vi "Main UI (standalone).vi"() -> ()   [LabVIEW 2015]
doc: "User interface for 64 pressure multiplexer system designed by Paul Nathan, 02/2016"
uses:
  Ctls/System status.ctl
  Ctls/Environmental state values.ctl
  Ctls/Inertial state values.ctl
  Ctls/AccelGyro constants.ctl
  Ctls/Pressure sensor constants.ctl
  Ctls/Cmd str.ctl
  Ctls/All state values (for datalog).ctl
  Ctls/Data values, Mode 0 (for datalog).ctl
  Ctls/Data values, Mode 1 (for datalog).ctl
panel:
  in  "Main tabs":enum32{"Startup & config.", "Datastream"}(tab)
  out "ASCII done":bool caption="Done"
  in  "Write ASCII datalog":bool
  in  "Datalog name (without extension)":string="Log001"
  in  "Write interval (s)":u32=10
  in  "Save data":bool
  in  "Datalog directory":path=path "C:/Datalogs"
  out "ACK 8":bool caption="ACK"
  out "ACK 7":bool caption="ACK"
  out "ACK 6":bool caption="ACK"
  out "AccelGyro constants":T1={"gyrRange"=125.0, "accRange"=2.0, "gx offset"=0.0, "gy offset"=0.0, "gz offset"=0.0, "ax offset"=0.0, "ay offset"=0.0, "az offset"=0.0, "axyz scale"=1.0} {"axyz scale" format="%#_4f"; "az offset" format="%#_4f"; "ay offset" format="%#_4f"; "ax offset" format="%#_4f"; "gz offset" format="%#_4f"; "gy offset" format="%#_4f"; "gx offset" format="%#_4f"; "gyrRange" format="%#_4f"; "accRange" format="%#_4f"}
  out "Faulty sensors":i32[](array[numeric])
  out "ACK 5":bool caption="ACK"
  in  "Stop UI":bool
  out "Active sensors":i32[](array[numeric])
  in  "Refresh sys. status":bool
  out "ACK 4":bool caption="ACK"
  in  "Apply settings 3":bool caption="Apply settings"
  in  "Gyro. rate (Hz)":u8(ring) items=["6.25", "12.5", "25", "50", "100", "200", "400", "800", "1600", "3200"]
  in  "Gyro. range (dps)":u8(ring) items=["+/- 125", "+/- 250", "+/- 500", "+/- 1000", "+/- 2000"]
  in  "Accel. rate (Hz)":u8(ring)=1 items=["3.125", "6.25", "12.5", "25", "50", "100", "200", "400", "800", "1600"]
  in  "Accel. range (g)":u8(ring) items=["+/- 2", "+/- 4", "+/- 8", "+/- 16"]
  out "Inertial state values":T2 {"w_z (dps)" format="%#_4f"; "a_y (g)" format="%#_4f"; "a_z (g)" format="%#_4f"; "w_y (dps)" format="%#_4f"; "a_x (g)" format="%#_4f"; "Sensor temp. (degC)" format="%#.2f"; "w_x (dps)" format="%#_4f"}
  out "Environmental state values":T3 {"Dew point (degC)" format="%#.2f"; "Density (kg/m^3)" format="%#.3f"; "Pressure alt. (m)" format="%#.2f"; "Density alt. (m)" format="%#.2f"; "Rel. Humidity (%)" format="%#.2f"; "P_atmos (Pa)" format="%#_6f"; "Sensor temp. (degC)" format="%#.2f"; "Thermistor (degC)" format="%#.2f"}
  out "System status":T4
  out "ACK 3":bool caption="ACK"
  in  "Apply settings 2":bool caption="Apply setting"
  in  "Max. num. sensors (override)":u8=64 max=64
  out "ACK 1":bool caption="ACK"
  in  "Env. period (ms)":i32=1000 min=0
  in  "Data mode":u8(ring) items=["P", "P & T"]
  out "ACK 2":bool caption="ACK"
  in  "Apply settings 1":bool caption="Apply settings"
  in  "Data rate (Hz)":dbl=100.0
  in  "Reset":bool
  in  "Main Power":bool
  in  "Serial port":refnum<visa-resource-name>="COM1"
  out "Error":errorcluster
  out "L_data (bytes)":u16
  out "Serial no.":u16 format="%04x"
  out "Active pressure sensor constants":T5[](array[typedef])
  in  "d.p":i16=4
  in  "Wait for HW trigger":bool
  out "Clock drift":bool
  in  "Display rate (Hz)":dbl=100.0 min=0.0
  in  "N samples":u32=1000
  in  "Finite samples":bool
  out "Sensor temperatures time trace (Mode \"P & T\" only)":sgl[][](graph)
  out "Pressures time trace":sgl[][](graph)
  in  "Stop streaming":bool
  in  "Start streaming":bool
  out "Stale samples flag":u8[][](graph)
  out "Samples acquired":u32
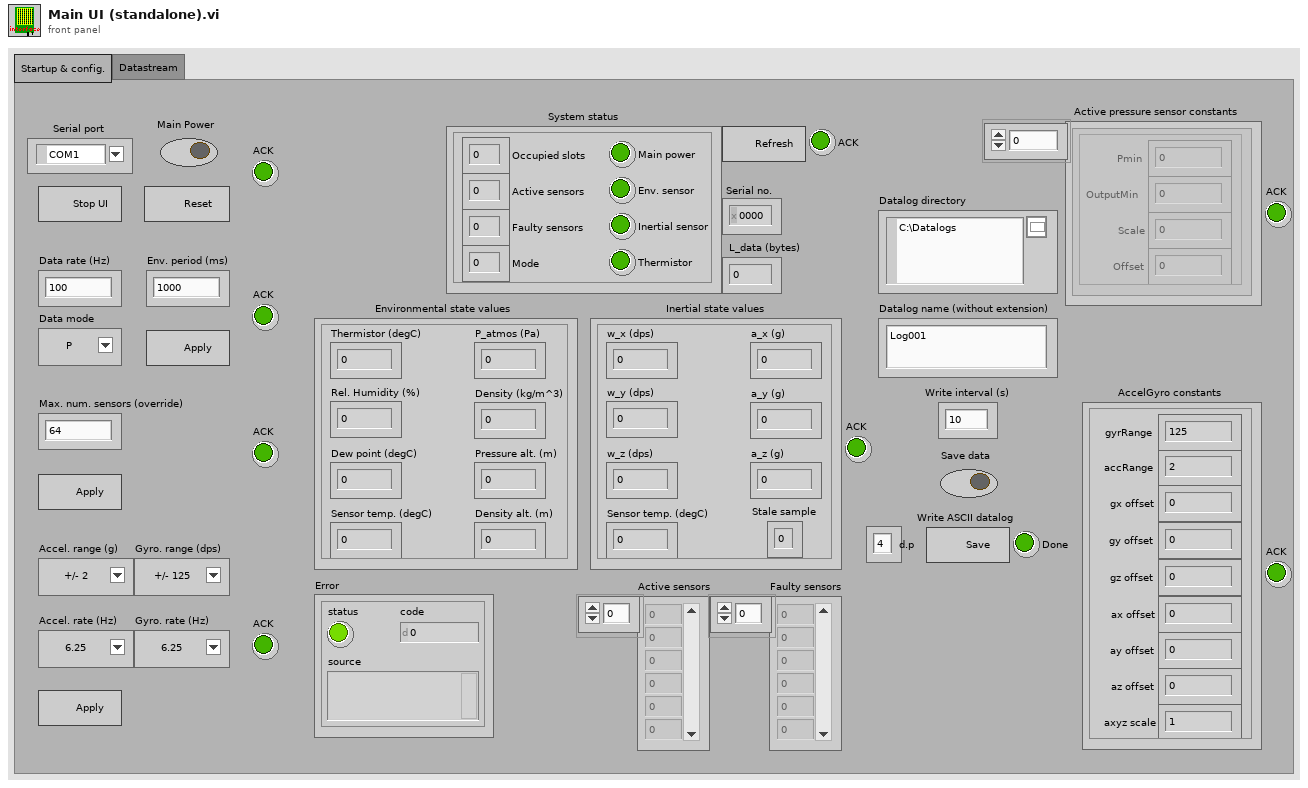
[diagram p1: front panel]
types:
  T1 = typedef "AccelGyro constants.ctl" = cluster{"gyrRange":sgl, "accRange":sgl, "gx offset":sgl, "gy offset":sgl, "gz offset":sgl, "ax offset":sgl, "ay offset":sgl, "az offset":sgl, "axyz scale":sgl}
  T2 = typedef "Inertial state values.ctl" = cluster{"w_x (dps)":sgl, "w_y (dps)":sgl, "w_z (dps)":sgl, "a_x (g)":sgl, "a_y (g)":sgl, "a_z (g)":sgl, "Stale sample":u8, "Sensor temp. (degC)":sgl}
  T3 = typedef "Environmental state values.ctl" = cluster{"Thermistor (degC)":sgl, "Sensor temp. (degC)":sgl, "P_atmos (Pa)":sgl, "Rel. Humidity (%)":sgl, "Density (kg/m^3)":sgl, "Dew point (degC)":sgl, "Pressure alt. (m)":sgl, "Density alt. (m)":sgl}
  T4 = typedef "System status.ctl" = cluster{"Main power":bool, "Occupied slots":u8, "Active sensors":u8, "Faulty sensors":u8, "Env. sensor":bool, "Inertial sensor":bool, "Thermistor":bool, "Mode":u8}
  T5 = typedef "Pressure sensor constants.ctl" = cluster{"Pmin":sgl, "OutputMin":sgl, "Scale":sgl, "Offset":sgl}
  T6 = typedef "Cmd str.ctl" = string
  T7 = typedef "All state values (for datalog).ctl" = cluster{"Time Stamp":timestamp, "dt (ms)":i32, "Environmental state values":T3, "Inertial state values":T2}
  T8 = typedef "Data values, Mode 1 (for datalog).ctl" = cluster{"Time Stamp":timestamp, "dt (us)":sgl, "dt_warn":u8, "Pressures":sgl[], "Die temps.":sgl[], "Statuses":u8[]}
  T9 = typedef "Data values, Mode 0 (for datalog).ctl" = cluster{"Time Stamp":timestamp, "dt (us)":sgl, "dt_warn":u8, "Pressures":sgl[], "Statuses":u8[]}
  T10 = enum8{"Enabled", "Disabled", "Disabled and Grayed Out"}
  T11 = typedef "EEPROM page.ctl" = cluster{"Pmin (Pa)":sgl, "Pmax (Pa)":sgl, "maxCount":u16, "minCount":u16, "Poffset (Pa)":sgl}
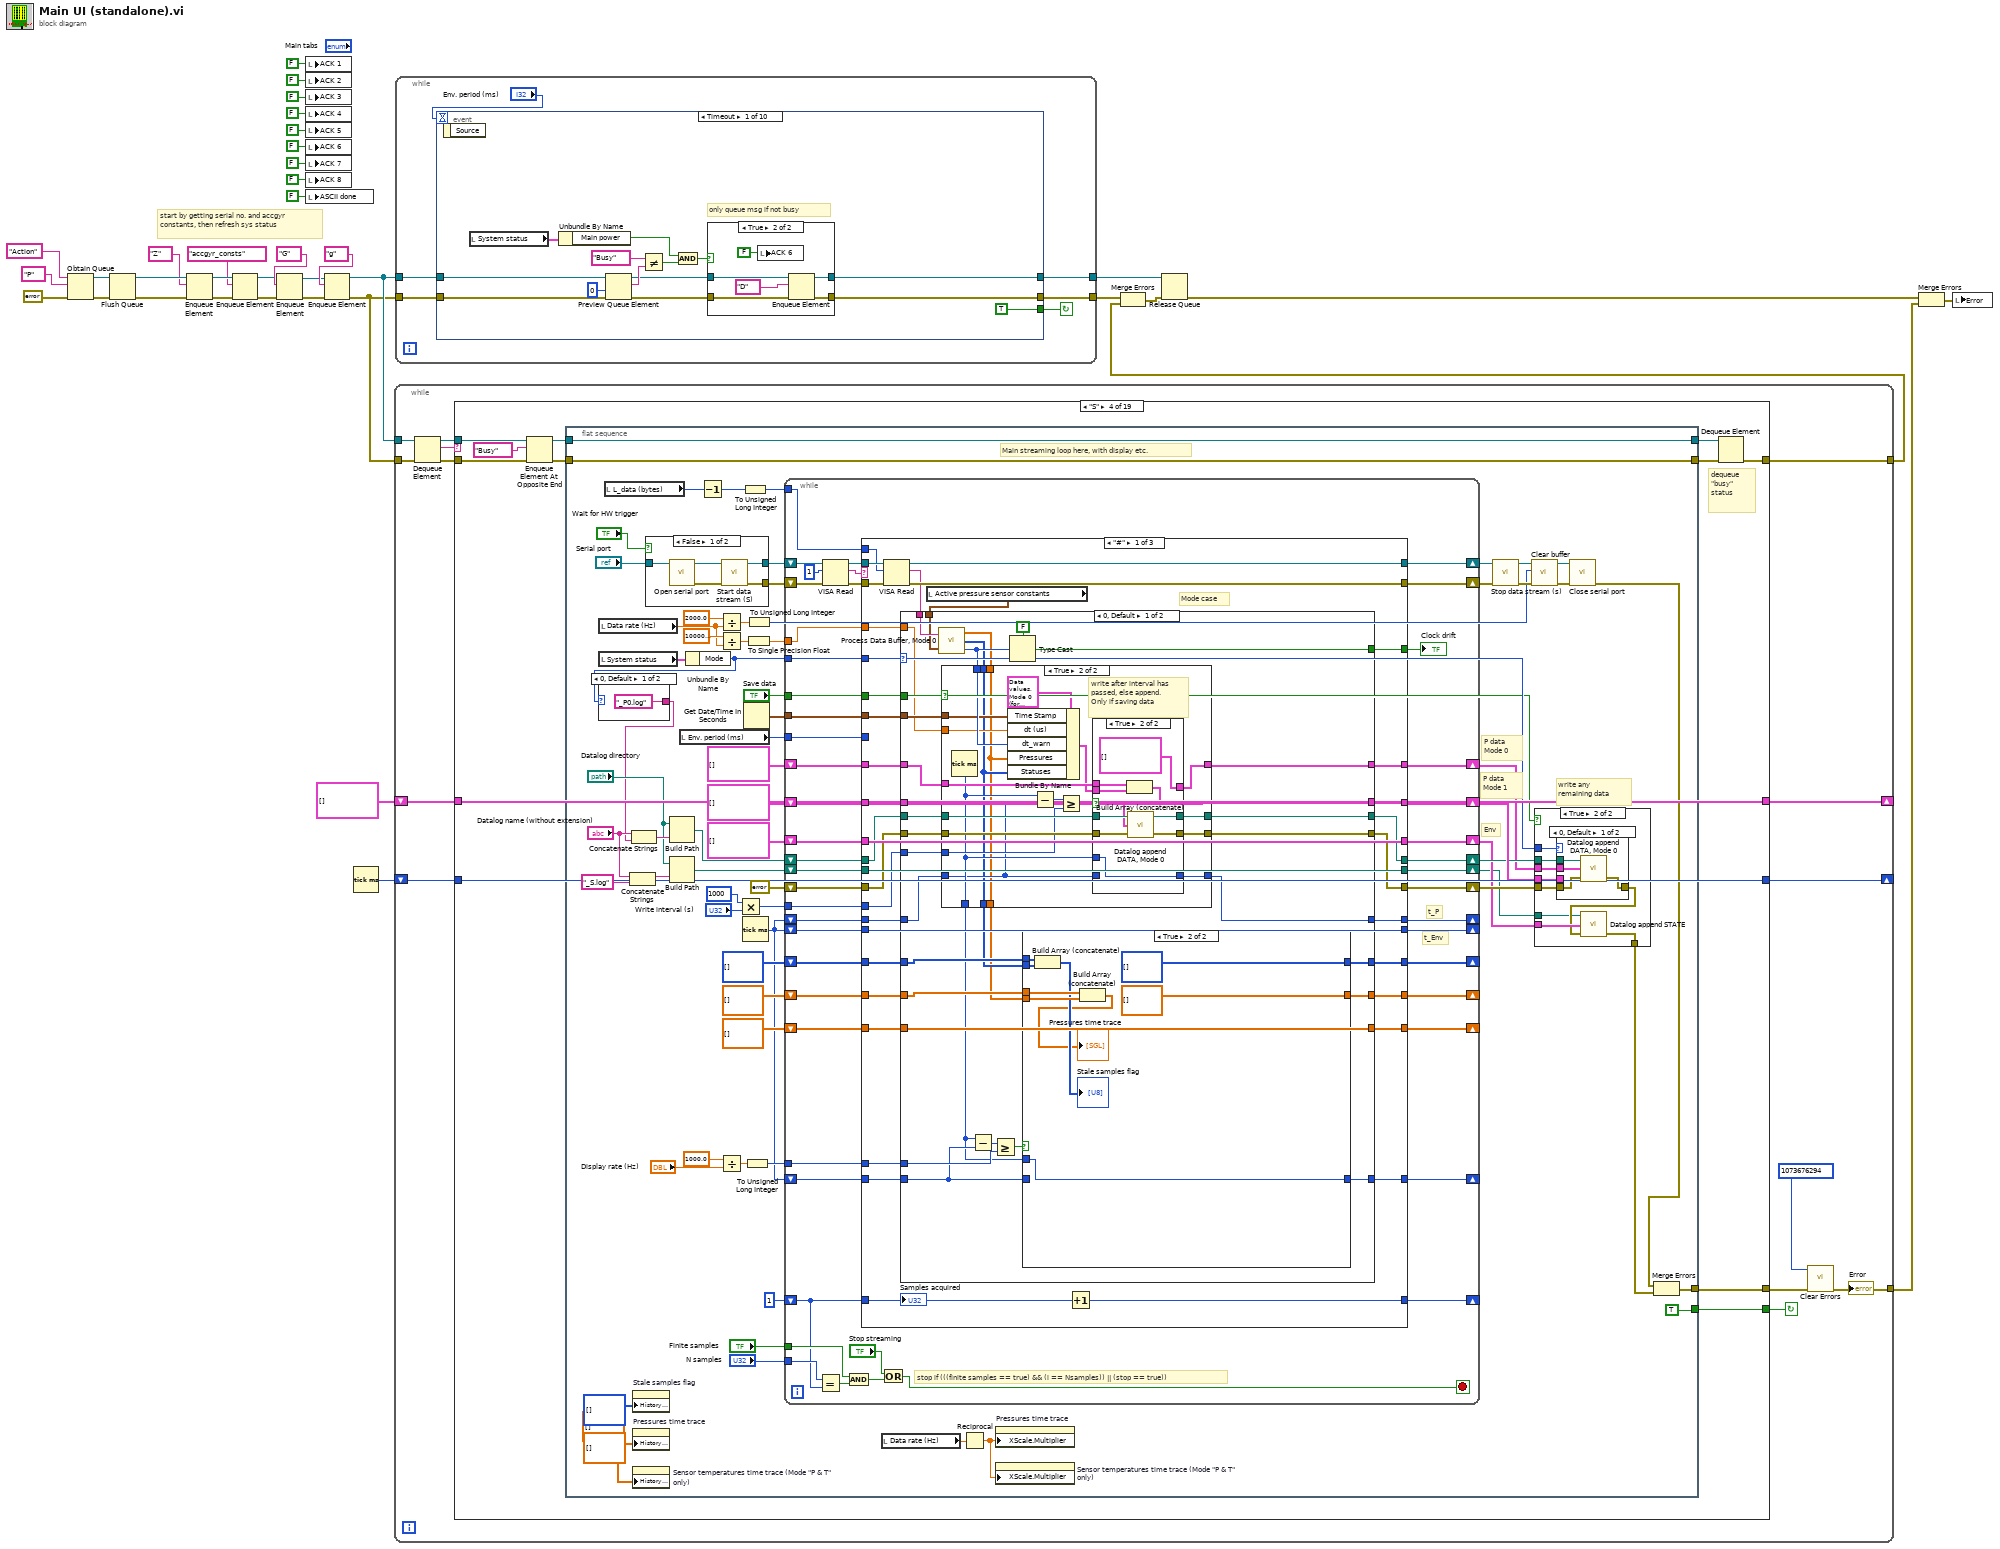
[diagram p0: block diagram]
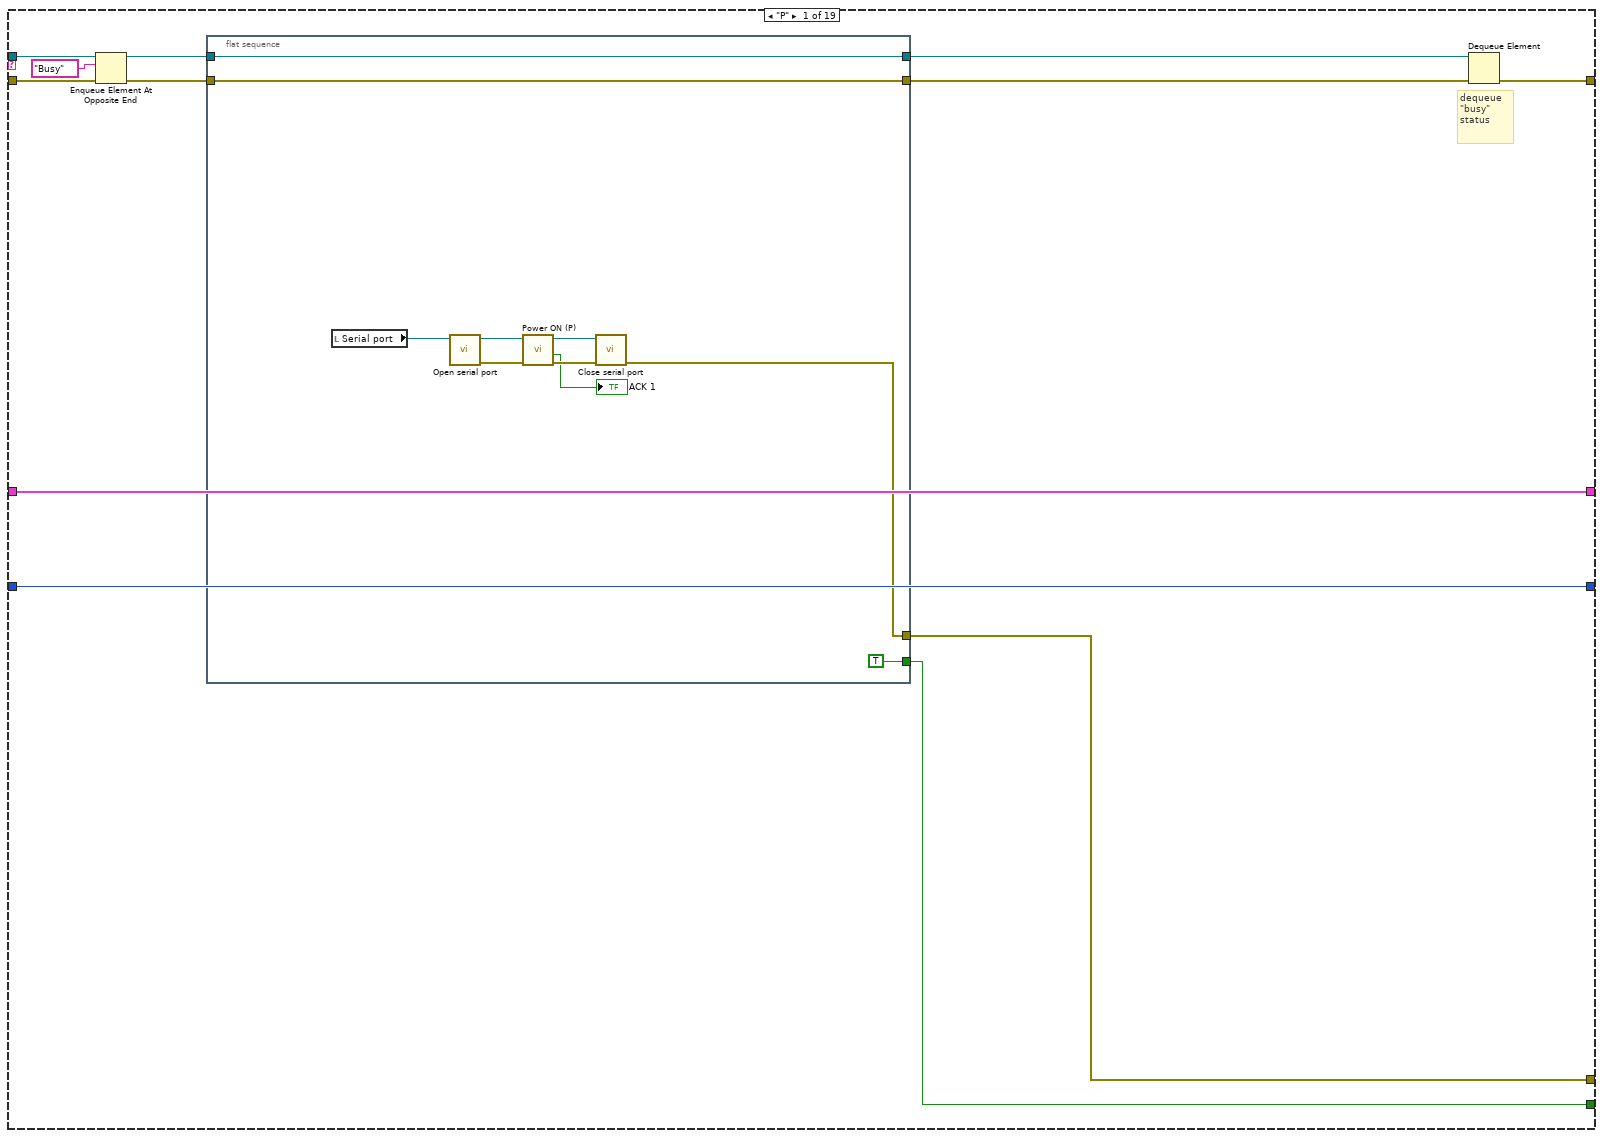
[diagram p2: hidden frame]
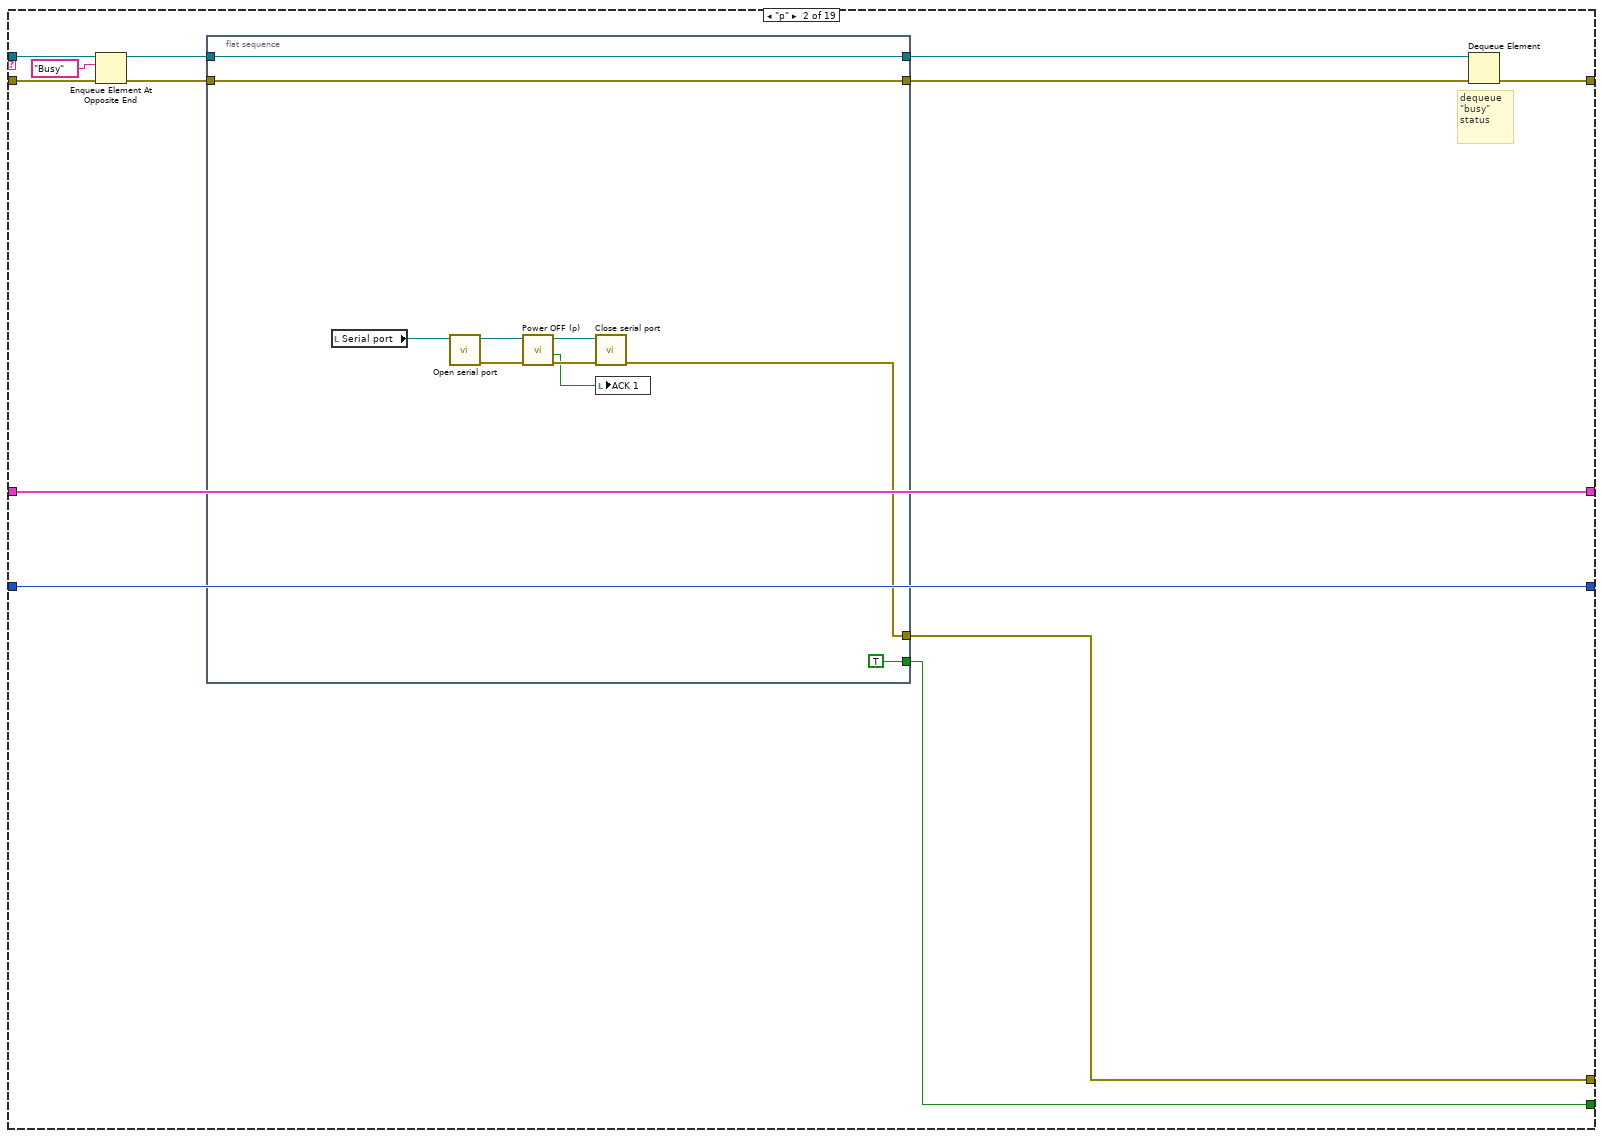
[diagram p3: hidden frame]
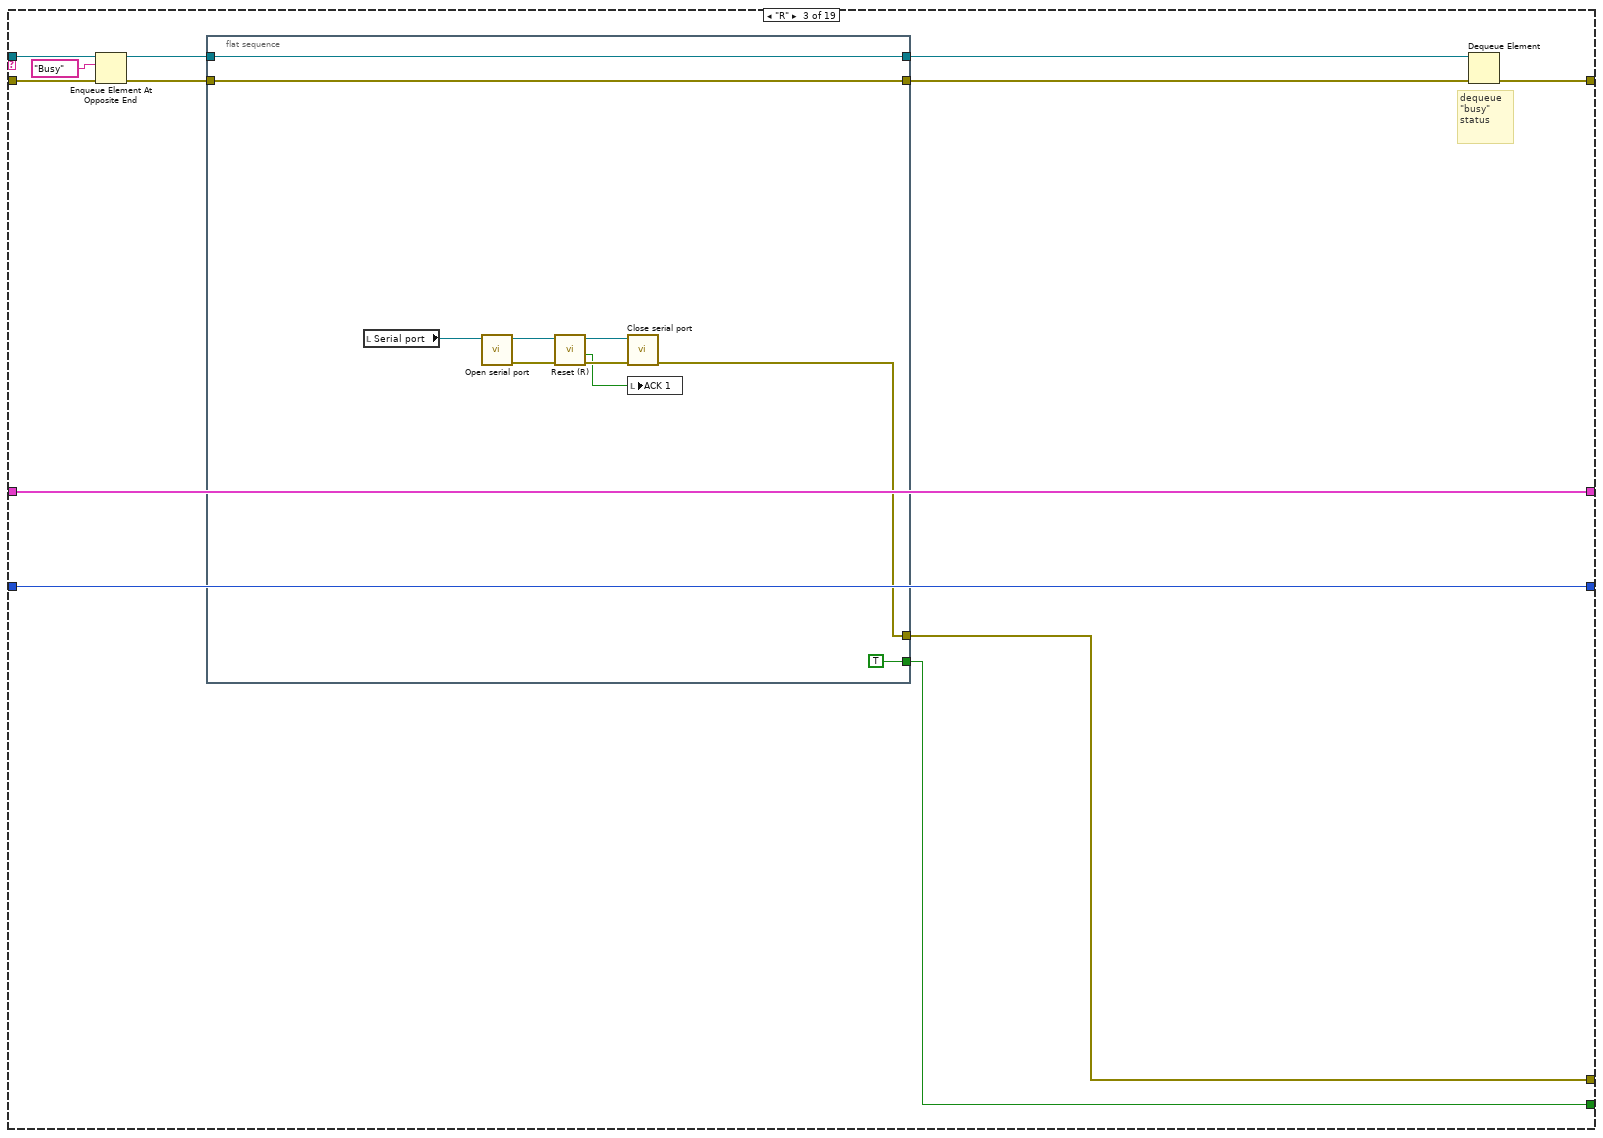
[diagram p4: hidden frame]
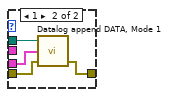
[diagram p6: hidden frame]
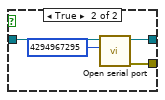
[diagram p7: hidden frame]
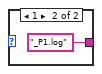
[diagram p8: hidden frame]
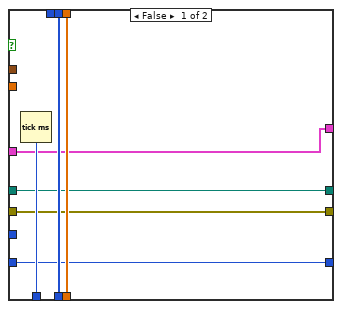
[diagram p9: hidden frame]
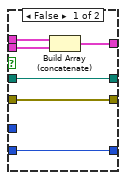
[diagram p10: hidden frame]
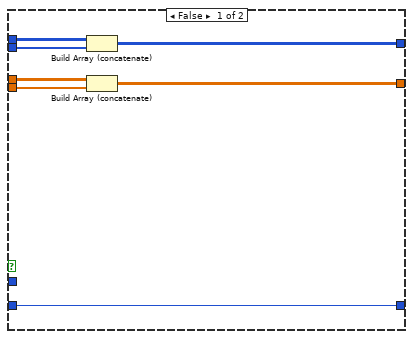
[diagram p11: hidden frame]
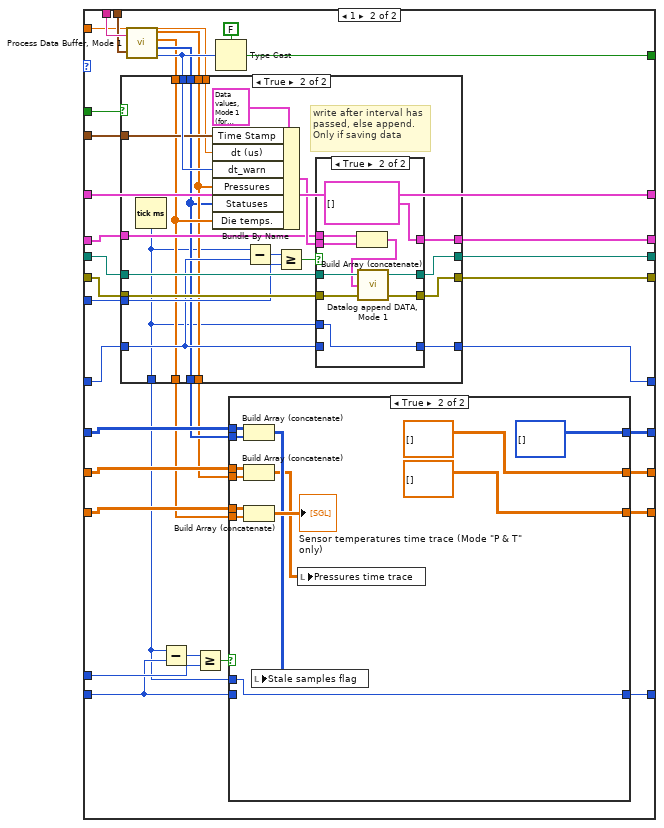
[diagram p12: hidden frame]
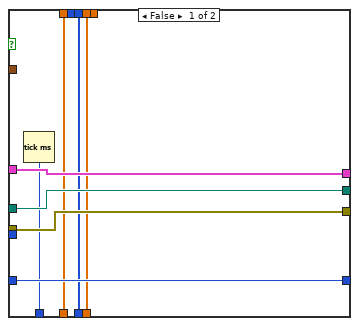
[diagram p13: hidden frame]
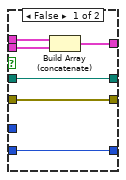
[diagram p14: hidden frame]
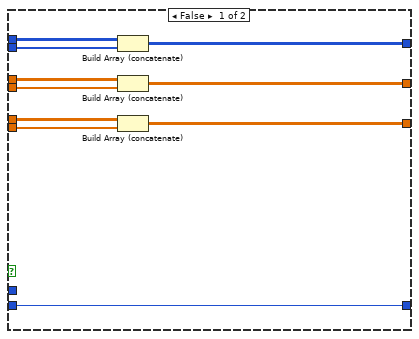
[diagram p15: hidden frame]
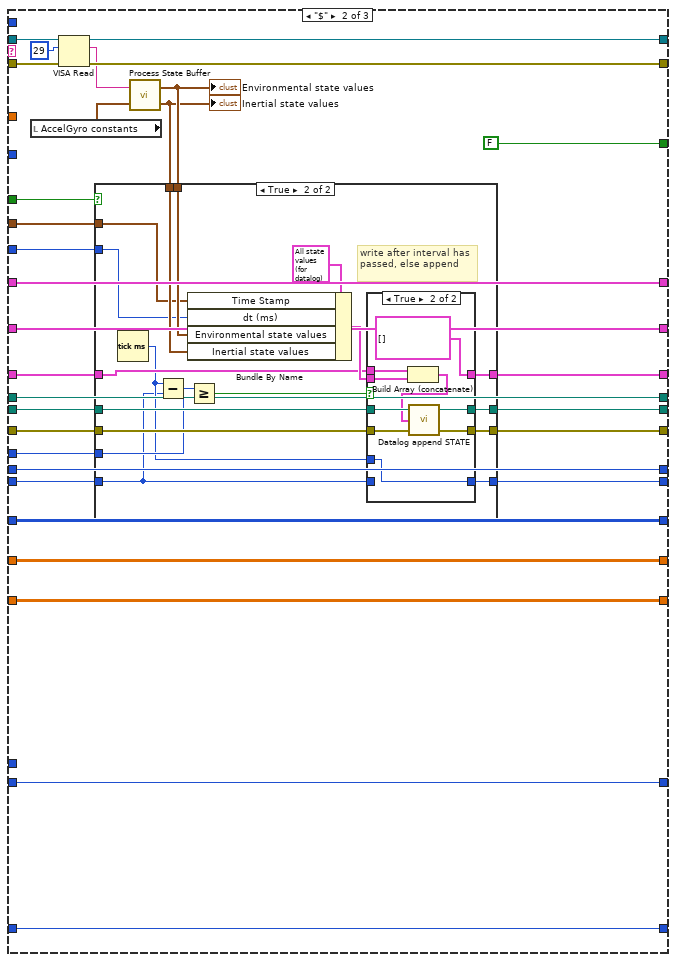
[diagram p16: hidden frame]
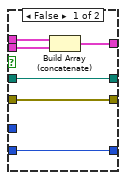
[diagram p18: hidden frame]
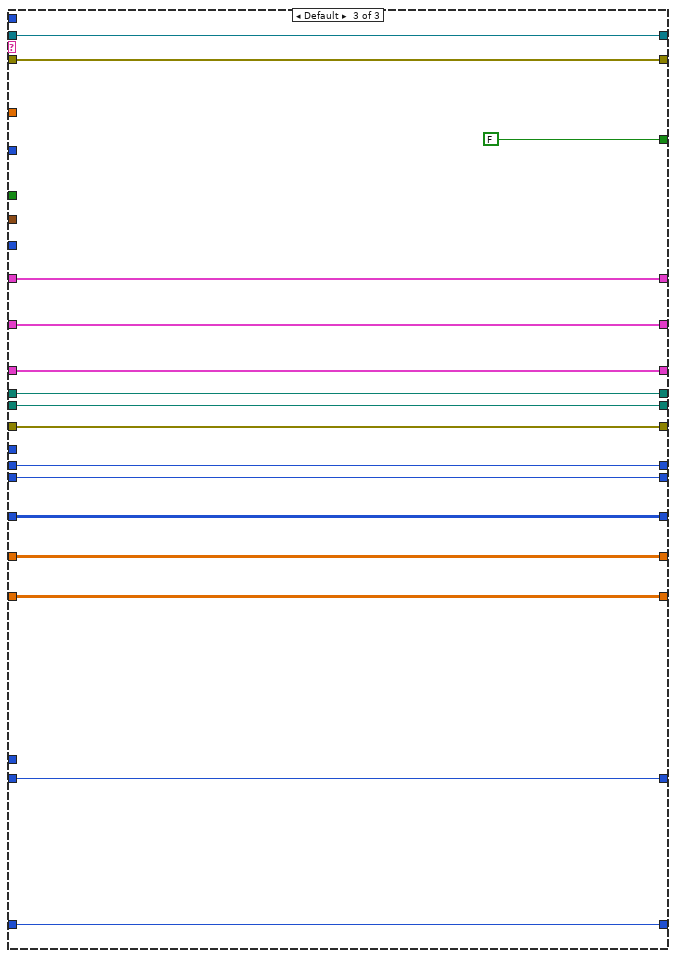
[diagram p19: hidden frame]
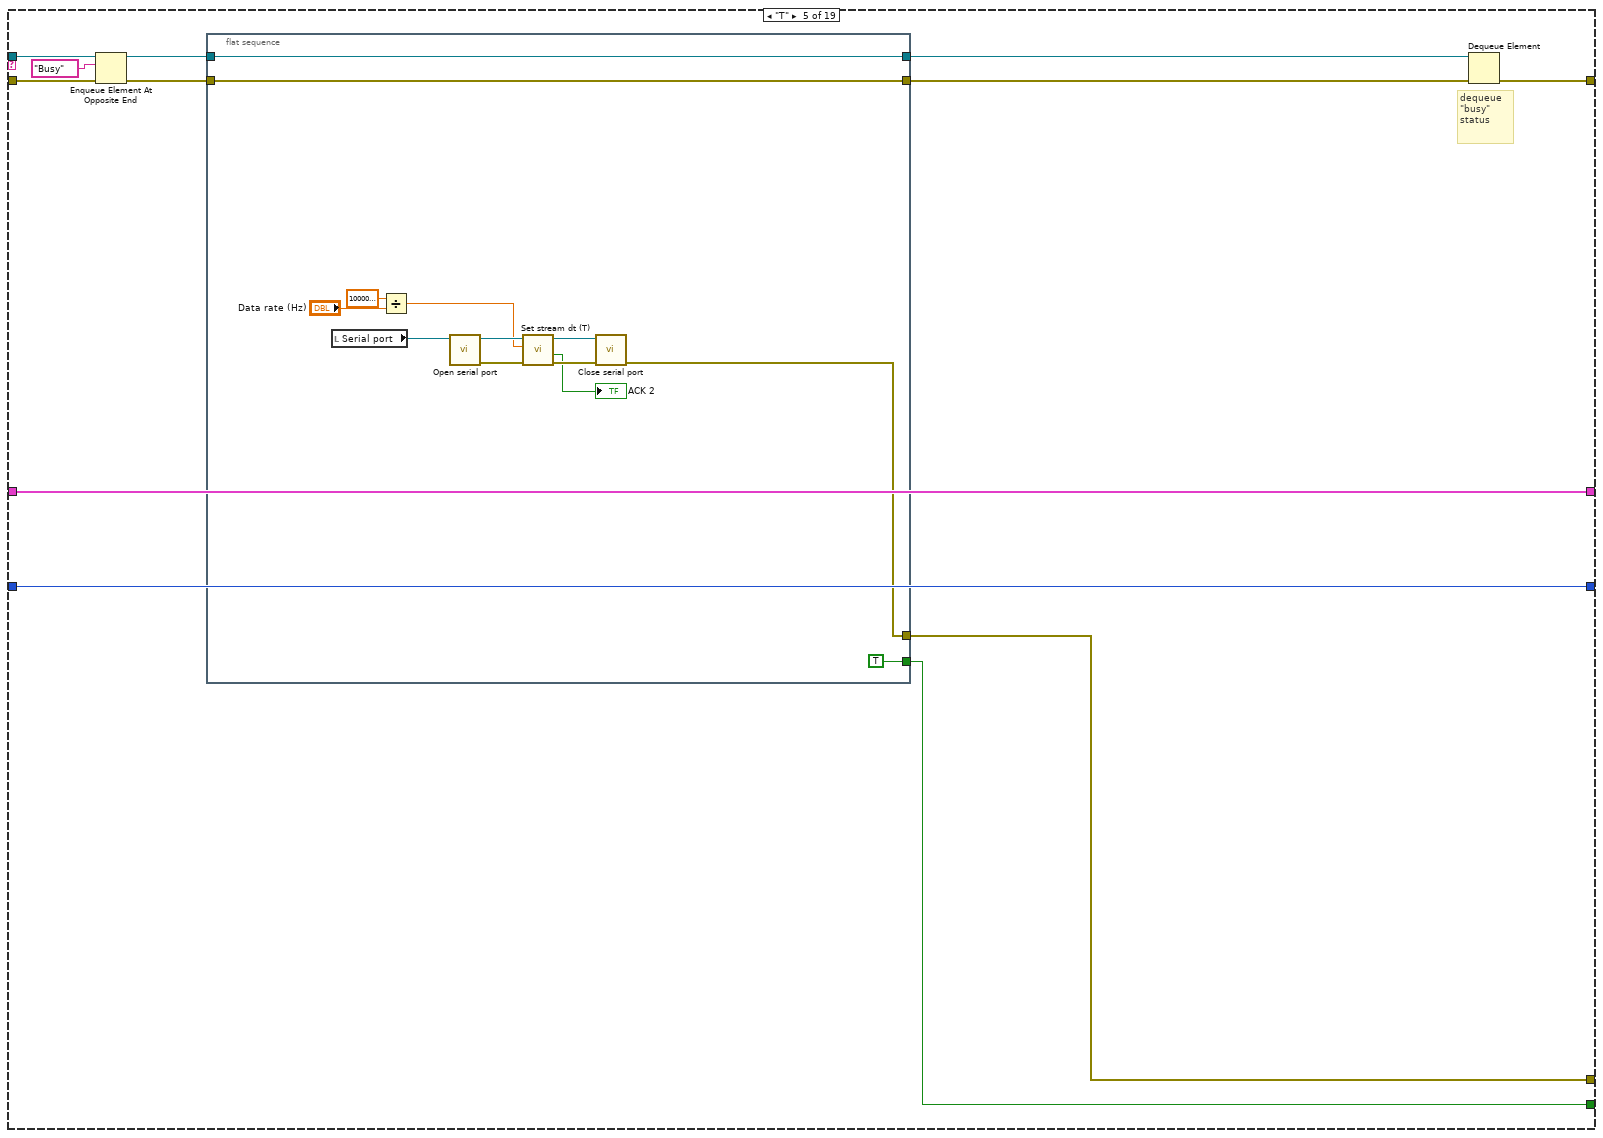
[diagram p20: hidden frame]
diagram:
  # "start by getting serial no. and accgyr constants, then refresh sys status"
  n1 = Obtain Queue(name (unnamed)="Action", element data type=T6 "P" ("Cmd"), error in (no error)=errorcluster {"status"=FALSE, "code"=0, "source"=""}) -> (queue out=w36:refnum<queue>, error out=w35:errorcluster)  [unwired: 2 in, 1 out]
  n2 = Flush Queue(queue=w36, error in (no error)=w35) -> (queue out=w28:refnum<queue>, error out=w27:errorcluster)  [unwired: 1 out]
  n3 = Enqueue Element(queue=w28, element=T6 "Z", error in (no error)=w27) -> (queue out=w25:refnum<queue>, error out=w24:errorcluster)  [unwired: 1 in, 1 out]
  n4 = Enqueue Element(queue=w25, element=T6 "accgyr_consts", error in (no error)=w24) -> (queue out=w12:refnum<queue>, error out=w11:errorcluster)  [unwired: 1 in, 1 out]
  n5 = Enqueue Element(queue=w12, element=T6 "G" ("Cmd"), error in (no error)=w11) -> (queue out=w14:refnum<queue>, error out=w15:errorcluster)  [unwired: 1 in, 1 out]
  n6 = local write "ACK 1"(FALSE ("ACK 8")) -> ()
  n7 = local write "ACK 2"(FALSE ("ACK 6")) -> ()
  n8 = local write "ACK 3"(FALSE ("ACK 8")) -> ()
  n9 = local write "ACK 4"(FALSE ("Done")) -> ()
  n10 = local write "ACK 5"(FALSE ("ACK 8")) -> ()
  n11 = local write "ACK 6"(FALSE ("ACK 6")) -> ()
  n12 = local write "ACK 7"(FALSE ("ACK 6")) -> ()
  n13 = local write "ACK 8"(FALSE ("ACK 8")) -> ()
  n14 = local write "ASCII done"(FALSE ("Done")) -> ()
  n15 = Enqueue Element(queue=w14, element=T6 "g" ("Cmd"), error in (no error)=w15) -> (queue out=w10:refnum<queue>, error out=w9:errorcluster)  [unwired: 1 in, 1 out]
  n16 = Tick Count (ms)() -> (millisecond timer value=w20:u32)
  n17 = while {
    tunnel: w9 -> [w50]
    tunnel: w10 -> [w51]
    tunnel: [w47] -> w30
    shift-right: [w44] -> _
    shift-left: T7[] [] -> [w43]
    tunnel: [w38] -> w18
    shift-right: [w41] -> _
    shift-left: w20 -> [w42]
    stop <- w46 continue-if-true
    n18 = Dequeue Element(queue=w51, error in (no error)=w50) -> (queue out=w49:refnum<queue>, element=w45:T6, error out=w48:errorcluster)  [unwired: 1 in, 1 out]
    n19 = case shown="\"S\"" w45 {
      tunnel: w49 -> [w63 w85 w107 w129 w600 w625 w649 w673 w697 w725 w762 w784 w806 w845 w869 w942 w974 w1002 _]
      tunnel: w48 -> [w62 w84 w106 w128 w599 w624 w648 w672 w696 w724 w761 w783 w805 w844 w868 w941 w973 w1001 w1071]
      tunnel: [w57 w79 w101 w123 w594 w619 w643 w667 w691 w719 w756 w778 w800 w839 w863 w936 w968 w996 w1071] -> w47
      tunnel: [w56 w78 w100 w122 w593 w618 w642 w666 w690 w718 w755 w777 w799 w838 w862 w935 w967 w995 FALSE] -> w46
      tunnel: [w55 w77 w99 w121 w592 w617 w641 w665 w689 w717 w754 w776 w798 w837 w861 w934 w966 w994 errorcluster {"status"=FALSE, "code"=0, "source"=""} ("Error out")] -> w39
      tunnel: [w53 w75 w97 w118 w590 w615 w639 w663 w687 w715 w752 w774 w796 w835 w859 w931 w964 w992 w1068] -> w44
      tunnel: w43 -> [w53 w75 w97 w118 w590 w615 w639 w663 w687 w715 w752 w774 w796 w835 w858 w931 w964 w992 w1068]
      tunnel: w42 -> [w52 w74 w96 w119 w589 w614 w638 w662 w686 w714 w751 w773 w795 w834 w857 w932 w963 w991 w1067]
      tunnel: [w52 w74 w96 w119 w589 w614 w638 w662 w686 w714 w751 w773 w795 w834 w856 w932 w963 w991 w1067] -> w41
      frame "P" {
        # "dequeue \"busy\" status"
        n20 = Enqueue Element At Opposite End(queue=w63, element=T6 "Busy" ("Cmd"), error in (no error)=w62) -> (queue out=w61:refnum<queue>, error out=w60:errorcluster)  [unwired: 1 in, 1 out]
        n21 = flat-sequence {
          tunnel: w61 -> [w73]
          tunnel: w60 -> [w72]
          tunnel: [w73] -> w59
          tunnel: [w72] -> w58
          tunnel: [TRUE] -> w56
          tunnel: [w66] -> w55
          frame #0 {
            n22 = local read "Serial port"() -> (w65:refnum<visa-resource-name>)
            n23 = call "Open serial port.vi"("VISA resource name"=w65) -> ("Error out"=w69:errorcluster, "VISA resource name out"=w70:refnum<visa-resource-name>)  [unwired: 9 in]
            n24 = call "Power ON (P).vi"("Error In"=w69, "VISA resource name in"=w70) -> ("Error out"=w68:errorcluster, "ACK"=→"ACK 1":bool, "VISA resource name out"=w67:refnum<visa-resource-name>)  [unwired: 7 in]
            n25 = call "Close serial port.vi"("Error in"=w68, "VISA resource name"=w67) -> ("Error out"=w66:errorcluster)  [unwired: 9 in]
          }
        }
        n26 = Dequeue Element(queue=w59, error in (no error)=w58) -> (error out=w57:errorcluster)  [unwired: 1 in, 3 out]
      }
      frame "p" {
        # "dequeue \"busy\" status"
        n27 = Enqueue Element At Opposite End(queue=w85, element=T6 "Busy" ("Cmd"), error in (no error)=w84) -> (queue out=w83:refnum<queue>, error out=w82:errorcluster)  [unwired: 1 in, 1 out]
        n28 = flat-sequence {
          tunnel: w83 -> [w95]
          tunnel: w82 -> [w94]
          tunnel: [w95] -> w81
          tunnel: [w94] -> w80
          tunnel: [TRUE] -> w78
          tunnel: [w88] -> w77
          frame #0 {
            n29 = local read "Serial port"() -> (w86:refnum<visa-resource-name>)
            n30 = call "Open serial port.vi"("VISA resource name"=w86) -> ("Error out"=w91:errorcluster, "VISA resource name out"=w92:refnum<visa-resource-name>)  [unwired: 9 in]
            n31 = call "Power OFF (p).vi"("Error In"=w91, "VISA resource name in"=w92) -> ("Error out"=w90:errorcluster, "ACK"=w87:bool, "VISA resource name out"=w89:refnum<visa-resource-name>)  [unwired: 7 in]
            n32 = call "Close serial port.vi"("Error in"=w90, "VISA resource name"=w89) -> ("Error out"=w88:errorcluster)  [unwired: 9 in]
            n33 = local write "ACK 1"(w87) -> ()
          }
        }
        n34 = Dequeue Element(queue=w81, error in (no error)=w80) -> (error out=w79:errorcluster)  [unwired: 1 in, 3 out]
      }
      frame "R" {
        # "dequeue \"busy\" status"
        n35 = Enqueue Element At Opposite End(queue=w107, element=T6 "Busy" ("Cmd"), error in (no error)=w106) -> (queue out=w105:refnum<queue>, error out=w104:errorcluster)  [unwired: 1 in, 1 out]
        n36 = flat-sequence {
          tunnel: w105 -> [w117]
          tunnel: w104 -> [w116]
          tunnel: [w117] -> w103
          tunnel: [w116] -> w102
          tunnel: [TRUE] -> w100
          tunnel: [w112] -> w99
          frame #0 {
            n37 = local read "Serial port"() -> (w110:refnum<visa-resource-name>)
            n38 = call "Open serial port.vi"("VISA resource name"=w110) -> ("Error out"=w108:errorcluster, "VISA resource name out"=w109:refnum<visa-resource-name>)  [unwired: 9 in]
            n39 = call "Reset (R).vi"("Error In"=w108, "VISA resource name in"=w109) -> ("Error out"=w114:errorcluster, "ACK"=w111:bool, "VISA resource name out"=w113:refnum<visa-resource-name>)  [unwired: 7 in]
            n40 = call "Close serial port.vi"("Error in"=w114, "VISA resource name"=w113) -> ("Error out"=w112:errorcluster)  [unwired: 9 in]
            n41 = local write "ACK 1"(w111) -> ()
          }
        }
        n42 = Dequeue Element(queue=w103, error in (no error)=w102) -> (error out=w101:errorcluster)  [unwired: 1 in, 3 out]
      }
      frame "S" {
        # "dequeue \"busy\" status"
        n43 = Enqueue Element At Opposite End(queue=w129, element=T6 "Busy" ("Cmd"), error in (no error)=w128) -> (queue out=w127:refnum<queue>, error out=w126:errorcluster)  [unwired: 1 in, 1 out]
        n44 = flat-sequence {
          tunnel: w127 -> [w197]
          tunnel: w126 -> [w196]
          tunnel: [w197] -> w125
          tunnel: [w196] -> w124
          tunnel: [TRUE] -> w122
          tunnel: [w183] -> w121
          frame #0 {
            # "Env"
            # "P data Mode 1"
            # "P data Mode 0"
            # "write any remaining data"
            # "Main streaming loop here, with display etc."
            n45 = local read "Data rate (Hz)"() -> (w158:dbl)
            n46 = local read "System status"() -> (w155:T4)
            n47 = local read "L_data (bytes)"() -> (w162:u16)
            n48 = Concatenate Strings("Datalog name (without extension)", "_S.log" ("string")) -> (w169:string)
            n49 = property on="Stale samples flag" class="WFChart (strict)"("History Data"=u8[][] []) -> ()  [unwired: 2 in, 2 out]
            n50 = property on="Pressures time trace" class="WFChart (strict)"("History Data"=sgl[][] []) -> ()  [unwired: 2 in, 2 out]
            n51 = property on="Sensor temperatures time trace (Mode \"P & T\" only)" class="WFChart (strict)"("History Data"=sgl[][] []) -> ()  [unwired: 2 in, 2 out]
            n52 = case shown="False" "Wait for HW trigger" {
              tunnel: [w218 w222] -> w194
              tunnel: [w217 w223] -> w193
              tunnel: "Serial port" -> [w216 w224]
              frame False {
                n53 = call "Open serial port.vi"("VISA resource name"=w216) -> ("Error out"=w219:errorcluster, "VISA resource name out"=w220:refnum<visa-resource-name>)  [unwired: 9 in]
                n54 = call "Start data stream (S).vi"("VISA resource name in"=w220, "Error In"=w219) -> ("VISA resource name out"=w217:refnum<visa-resource-name>, "Error out"=w218:errorcluster)  [unwired: 7 in]
              }
              frame True {
                n55 = call "Open serial port.vi"("timeout (ms)"=u32 4294967295, "VISA resource name"=w224) -> ("Error out"=w222:errorcluster, "VISA resource name out"=w223:refnum<visa-resource-name>)  [unwired: 8 in]
              }
            }
            n56 = Build Path(base path="Datalog directory", name or relative path=w169) -> (appended path=w165:path)
            n57 = local read "Env. period (ms)"() -> (w160:i32)
            n58 = Unbundle By Name(w155) -> ("Mode"=w140:u8)
            n59 = case shown="0, Default" w140 {
              tunnel: ["_P0.log" ("string") "_P1.log" ("string")] -> w154
              frame 0, Default {
              }
              frame 1 {
              }
            }
            n60 = Concatenate Strings("Datalog name (without extension)", w154) -> (w177:string)
            n61 = Build Path(base path="Datalog directory", name or relative path=w177) -> (appended path=w166:path)
            n62 = Decrement(x=w162) -> (x-1=w144:u16)
            n63 = Divide(x=2000.0 ("y"), y=w158) -> (x/y=w186:dbl)
            n64 = Divide(x=1000000.0 ("y"), y=w158) -> (x/y=w157:dbl)
            n65 = Divide(x=1000.0, y="Display rate (Hz)") -> (x/y=w175:dbl)
            n66 = Multiply(x=u32 1000, y="Write interval (s)") -> (x*y=w179:u32)
            n67 = To Unsigned Long Integer(number=w144) -> (unsigned 32bit integer=w161:u32)
            n68 = Tick Count (ms)() -> (millisecond timer value=w145:u32)
            n69 = Get Date/Time In Seconds() -> (seconds since 1Jan1904=w192:timestamp)
            n70 = To Unsigned Long Integer(number=w175) -> (unsigned 32bit integer=w172:u32)
            n71 = To Unsigned Long Integer(number=w186) -> (unsigned 32bit integer=w185:u32)
            n72 = To Single Precision Float(number=w157) -> (single precision float=w156:sgl)
            n73 = while {
              shift-right: [w269] -> w189
              shift-left: w193 -> [w274]
              shift-right: [w268] -> w190
              shift-left: w194 -> [w275]
              tunnel: w192 -> [w267]
              shift-right: [w266] -> w142
              shift-left: errorcluster {"status"=FALSE, "code"=0, "source"=""} ("Error out") -> [w265]
              tunnel: "Finite samples" -> [w262]
              tunnel: "N samples" -> [w264]
              tunnel: "Save data" -> [w258]
              shift-right: [w256] -> w136
              shift-left: w165 -> [w257]
              shift-right: [w255] -> w138
              shift-left: T7[] [] -> [w254]
              tunnel: w179 -> [w252]
              shift-right: [w247] -> _
              shift-left: w145 -> [w253]
              tunnel: w172 -> [w236]
              shift-right: [w250] -> w141
              shift-left: w166 -> [w251]
              shift-right: [w248] -> _
              shift-left: w145 -> [w249]
              shift-right: [w243] -> w143
              shift-left: T8[] [] -> [w245]
              shift-right: [w244] -> w139
              shift-left: T9[] [] -> [w246]
              tunnel: w161 -> [w242]
              tunnel: w160 -> [w241]
              tunnel: w156 -> [w240]
              tunnel: w140 -> [w229]
              shift-right: [w238] -> _
              shift-left: w145 -> [w237]
              shift-right: [w235] -> _
              shift-left: sgl[][] [] -> [w232]
              shift-right: [w234] -> _
              shift-left: u8[][] [] -> [w233]
              shift-right: [w231] -> _
              shift-left: sgl[][] [] -> [w230]
              shift-right: [w228] -> _
              shift-left: u32 1 ("x") -> [w227]
              stop <- w259 stop-if-true
              # "t_Env"
              # "t_P"
              # "stop if (((finite samples == true) && (i == Nsamples)) || (stop == true))"
              n74 = Equal?(x=w264, y=w227) -> (x = y?=w263:bool)
              n75 = VISA Read(VISA resource name=w274, byte count=u32 1, error in (no error)=w275) -> (VISA resource name out=w271:refnum<visa-resource-name>, read buffer=w272:string, error out=w270:errorcluster)  [unwired: 1 out]
              n76 = And(x=w262, y=w263) -> (x .and. y?=w260:bool)
              n77 = case shown="\"#\"" w272 {
                tunnel: w271 -> [w310 w534 w588]
                tunnel: w270 -> [w309 w533 w587]
                tunnel: [w307 w531 w588] -> w269
                tunnel: [w306 w532 w587] -> w268
                tunnel: w267 -> [w303 w528 _]
                tunnel: [w289 w527 w586] -> w266
                tunnel: w265 -> [w299 w526 w586]
                tunnel: w258 -> [w278 w525 _]
                tunnel: w257 -> [w312 w524 w585]
                tunnel: [w312 w523 w585] -> w256
                tunnel: [w311 w522 w584] -> w255
                tunnel: w254 -> [w311 w521 w584]
                tunnel: w253 -> [w294 w514 w581]
                tunnel: w252 -> [w296 w520 _]
                tunnel: [w295 w519 w582] -> w248
                tunnel: w251 -> [w300 w516 w583]
                tunnel: [w288 w516 w583] -> w250
                tunnel: w249 -> [w295 w515 w582]
                tunnel: [w298 w514 w581] -> w247
                tunnel: w246 -> [w302 w513 w579]
                tunnel: w245 -> [w291 w512 w580]
                tunnel: [w301 w513 w579] -> w244
                tunnel: [w290 w512 w580] -> w243
                tunnel: w242 -> [w308 _ _]
                tunnel: w241 -> [_ w511 _]
                tunnel: w240 -> [w297 _ _]
                tunnel: [w293 FALSE ("Clock drift") FALSE ("Clock drift")] -> w239
                tunnel: w229 -> [w292 _ _]
                tunnel: [w287 w509 w577] -> w238
                tunnel: w237 -> [w286 w509 w577]
                tunnel: w236 -> [w285 _ _]
                tunnel: [w284 w507 w575] -> w235
                tunnel: w232 -> [w283 w507 w575]
                tunnel: [w282 w508 w576] -> w234
                tunnel: w233 -> [w281 w508 w576]
                tunnel: [w280 w506 w574] -> w231
                tunnel: w230 -> [w279 w506 w574]
                tunnel: [w277 w505 w573] -> w228
                tunnel: w227 -> [w276 w505 w573]
                frame "#" {
                  # "Mode case"
                  n78 = VISA Read(VISA resource name=w310, byte count=w308, error in (no error)=w309) -> (VISA resource name out=w307:refnum<visa-resource-name>, read buffer=w305:string, error out=w306:errorcluster)  [unwired: 1 out]
                  n79 = local read "Active pressure sensor constants"() -> (w304:T5[])
                  n80 = case shown="0, Default" w292 {
                    tunnel: w305 -> [w344 w437]
                    tunnel: w304 -> [w343 w436]
                    tunnel: w303 -> [w340 w433]
                    tunnel: w302 -> [w339 w438]
                    tunnel: [w338 w438] -> w301
                    tunnel: w300 -> [w337 w432]
                    tunnel: w299 -> [w336 w431]
                    tunnel: [w335 w430] -> w298
                    tunnel: w297 -> [w334 w429]
                    tunnel: w296 -> [w333 w428]
                    tunnel: w294 -> [w318 w427]
                    tunnel: [w332 w426] -> w293
                    tunnel: w291 -> [w345 w425]
                    tunnel: [w345 w424] -> w290
                    tunnel: [w313 w403] -> w289
                    tunnel: [w331 w423] -> w288
                    tunnel: [w330 w417] -> w287
                    tunnel: w286 -> [w327 w413]
                    tunnel: w285 -> [w329 w414]
                    tunnel: [w324 w421] -> w284
                    tunnel: w283 -> [w323 w419]
                    tunnel: [w321 w422] -> w282
                    tunnel: w281 -> [w320 w420]
                    tunnel: [w319 w411] -> w280
                    tunnel: w279 -> [w319 w409]
                    tunnel: w278 -> [w315 w408]
                    frame 0, Default {
                      n81 = call "Process Data Buffer, Mode 0.vi"("DATA_Buffer excluding '#' [1...N]"=w344, "P constants"=w343) -> ("Pressures"=w325:sgl[], "Statuses"=w322:u8[], "dt_warn"=w341:u8)
                      n82 = case shown="True" w315 {
                        tunnel: w341 -> [_ w370]
                        tunnel: w340 -> [_ w369]
                        tunnel: w339 -> [w347 w368]
                        tunnel: [w347 w366] -> w338
                        tunnel: w337 -> [w348 w365]
                        tunnel: w336 -> [w349 w364]
                        tunnel: [w346 w363] -> w335
                        tunnel: w334 -> [_ w362]
                        tunnel: w333 -> [_ w359]
                        tunnel: [w349 w358] -> w313
                        tunnel: [w348 w357] -> w331
                        tunnel: [w352 w356] -> w314
                        tunnel: w325 -> [w350 w353]
                        tunnel: w322 -> [w351 w354]
                        tunnel: w318 -> [w346 w355]
                        tunnel: [w351 w354] -> w317
                        tunnel: [w350 w353] -> w316
                        frame False {
                          n83 = Tick Count (ms)() -> (millisecond timer value=w352:u32)
                        }
                        frame True {
                          # "write after interval has passed, else append. Only if saving data"
                          n84 = Tick Count (ms)() -> (millisecond timer value=w356:u32)
                          n85 = Bundle By Name(cluster=T9 {"Time Stamp"=timestamp(3537581686.1176577 s since 1904-01-01), "dt (us)"=0.0, "dt_warn"=0, "Pressures"=[], "Statuses"=[]} ("P data (Mode 0)"), "Time Stamp"=w369, "dt (us)"=w362, "dt_warn"=w370, "Pressures"=w353, "Statuses"=w354) -> (w367:T9)
                          n86 = Subtract(x=w356, y=w355) -> (x-y=w361:u32)
                          n87 = Greater Or Equal?(x=w361, y=w359) -> (x >= y?=w360:bool)
                          n88 = case shown="True" w360 {
                            tunnel: [w373 w386] -> w358
                            tunnel: w364 -> [w373 w385]
                            tunnel: w365 -> [w374 w384]
                            tunnel: [w374 w383] -> w357
                            tunnel: w367 -> [w376 w382]
                            tunnel: w368 -> [w377 w381]
                            tunnel: [w375 T9[] []] -> w366
                            tunnel: w356 -> [_ w380]
                            tunnel: [w372 w380] -> w363
                            tunnel: w355 -> [w372 _]
                            frame False {
                              n89 = Build Array (concatenate)(w377, w376) -> (w375:T9[])
                            }
                            frame True {
                              n90 = Build Array (concatenate)(w381, w382) -> (w378:T9[])
                              n91 = call "Datalog append DATA, Mode 0.vi"("Datalog (Data) path"=w384, "Data (Mode 0)"=w378, "Error in"=w385) -> ("Path out"=w383:path, "Error out"=w386:errorcluster)  [unwired: 5 in]
                            }
                          }
                        }
                      }
                      n92 = Subtract(x=w314, y=w327) -> (x-y=w328:u32)
                      n93 = Greater Or Equal?(x=w328, y=w329) -> (x >= y?=w326:bool)
                      n94 = Type Cast(type=FALSE ("Clock drift"), x=w341) -> (*(type *) &x=w332:bool)
                      n95 = case shown="True" w326 {
                        tunnel: [w393 w402] -> w330
                        tunnel: w327 -> [w393 _]
                        tunnel: w314 -> [_ w402]
                        tunnel: w316 -> [w392 w400]
                        tunnel: [w391 sgl[][] []] -> w324
                        tunnel: w323 -> [w390 w401]
                        tunnel: w317 -> [w389 w397]
                        tunnel: [w388 u8[][] []] -> w321
                        tunnel: w320 -> [w387 w398]
                        frame False {
                          n96 = Build Array (concatenate)(w387, w389) -> (w388:u8[][])
                          n97 = Build Array (concatenate)(w390, w392) -> (w391:sgl[][])
                        }
                        frame True {
                          n98 = Build Array (concatenate)(w398, w397) -> (→"Stale samples flag":u8[][])
                          n99 = Build Array (concatenate)(w401, w400) -> (→"Pressures time trace":sgl[][])
                        }
                      }
                    }
                    frame 1 {
                      n100 = call "Process Data Buffer, Mode 1.vi"("DATA_Buffer excluding '#' [1...N]"=w437, "P constants"=w436) -> ("Pressures (Pa)"=w418:sgl[], "Sensor temps (degC)"=w410:sgl[], "Statuses"=w412:u8[], "dt_warn"=w434:u8)
                      n101 = case shown="True" w408 {
                        tunnel: w434 -> [_ w465]
                        tunnel: w433 -> [_ w464]
                        tunnel: w432 -> [w444 w462]
                        tunnel: w431 -> [w445 w461]
                        tunnel: [w446 w460] -> w430
                        tunnel: w429 -> [_ w459]
                        tunnel: w428 -> [_ w456]
                        tunnel: w427 -> [w446 w455]
                        tunnel: w425 -> [w443 w454]
                        tunnel: [w443 w453] -> w424
                        tunnel: [w445 w452] -> w403
                        tunnel: [w444 w451] -> w423
                        tunnel: w418 -> [w441 w449]
                        tunnel: w412 -> [w440 w448]
                        tunnel: w410 -> [w442 w450]
                        tunnel: [w442 w450] -> w407
                        tunnel: [w441 w449] -> w405
                        tunnel: [w440 w448] -> w406
                        tunnel: [w439 w447] -> w404
                        frame False {
                          n102 = Tick Count (ms)() -> (millisecond timer value=w439:u32)
                        }
                        frame True {
                          # "write after interval has passed, else append. Only if saving data"
                          n103 = Tick Count (ms)() -> (millisecond timer value=w447:u32)
                          n104 = Bundle By Name(cluster=T8 {"Time Stamp"=timestamp(3537581686.1176577 s since 1904-01-01), "dt (us)"=0.0, "dt_warn"=0, "Pressures"=[], "Die temps."=[], "Statuses"=[]} ("P data (Mode 1)"), "Time Stamp"=w464, "dt (us)"=w459, "dt_warn"=w465, "Pressures"=w449, "Statuses"=w448, "Die temps."=w450) -> (w463:T8)
                          n105 = Subtract(x=w447, y=w455) -> (x-y=w458:u32)
                          n106 = Greater Or Equal?(x=w458, y=w456) -> (x >= y?=w457:bool)
                          n107 = case shown="True" w457 {
                            tunnel: [w468 w481] -> w452
                            tunnel: w461 -> [w468 w480]
                            tunnel: w462 -> [w469 w479]
                            tunnel: [w469 w478] -> w451
                            tunnel: w463 -> [w471 w477]
                            tunnel: w454 -> [w472 w476]
                            tunnel: [w470 T8[] []] -> w453
                            tunnel: w447 -> [_ w475]
                            tunnel: [w467 w475] -> w460
                            tunnel: w455 -> [w467 _]
                            frame False {
                              n108 = Build Array (concatenate)(w472, w471) -> (w470:T8[])
                            }
                            frame True {
                              n109 = Build Array (concatenate)(w476, w477) -> (w474:T8[])
                              n110 = call "Datalog append DATA, Mode 1.vi"("Datalog (Data) path"=w479, "Data (Mode 1)"=w474, "Error in"=w480) -> ("Path out"=w478:path, "Error out"=w481:errorcluster)  [unwired: 5 in]
                            }
                          }
                        }
                      }
                      n111 = Subtract(x=w404, y=w413) -> (x-y=w416:u32)
                      n112 = Greater Or Equal?(x=w416, y=w414) -> (x >= y?=w415:bool)
                      n113 = Type Cast(type=FALSE ("Clock drift"), x=w434) -> (*(type *) &x=w426:bool)
                      n114 = case shown="True" w415 {
                        tunnel: [w491 w504] -> w417
                        tunnel: w413 -> [w491 _]
                        tunnel: w404 -> [_ w504]
                        tunnel: w405 -> [w490 w502]
                        tunnel: [w489 sgl[][] []] -> w421
                        tunnel: w419 -> [w488 w503]
                        tunnel: w406 -> [w487 w499]
                        tunnel: [w486 u8[][] []] -> w422
                        tunnel: w420 -> [w485 w500]
                        tunnel: [w484 sgl[][] []] -> w411
                        tunnel: w407 -> [w483 w495]
                        tunnel: w409 -> [w482 w496]
                        frame False {
                          n115 = Build Array (concatenate)(w485, w487) -> (w486:u8[][])
                          n116 = Build Array (concatenate)(w488, w490) -> (w489:sgl[][])
                          n117 = Build Array (concatenate)(w482, w483) -> (w484:sgl[][])
                        }
                        frame True {
                          n118 = Build Array (concatenate)(w500, w499) -> (w493:u8[][])
                          n119 = Build Array (concatenate)(w503, w502) -> (w492:sgl[][])
                          n120 = Build Array (concatenate)(w496, w495) -> (→"Sensor temperatures time trace (Mode \"P & T\" only)":sgl[][])
                          n121 = local write "Stale samples flag"(w493) -> ()
                          n122 = local write "Pressures time trace"(w492) -> ()
                        }
                      }
                    }
                  }
                  n123 = Increment(x=w276) -> (x+1=w277:u32)
                  "Samples acquired" <- w276
                }
                frame "$" {
                  n124 = local read "AccelGyro constants"() -> (w529:T1)
                  n125 = VISA Read(VISA resource name=w534, byte count=u32 29, error in (no error)=w533) -> (VISA resource name out=w531:refnum<visa-resource-name>, read buffer=w530:string, error out=w532:errorcluster)  [unwired: 1 out]
                  n126 = call "Process State Buffer.vi"("AccelGyro constants"=w529, "STATE_Buffer excluding '$' [1...30]"=w530) -> ("Inertial state values"=w517:T2, "Environmental state values"=w518:T3)
                  "Environmental state values" <- w518
                  "Inertial state values" <- w517
                  n127 = case shown="True" w525 {
                    tunnel: w518 -> [_ w556]
                    tunnel: w517 -> [_ w555]
                    tunnel: w528 -> [_ w554]
                    tunnel: [w539 w553] -> w527
                    tunnel: w526 -> [w539 w552]
                    tunnel: w524 -> [w538 w551]
                    tunnel: [w538 w550] -> w523
                    tunnel: [w537 w548] -> w522
                    tunnel: w521 -> [w537 w547]
                    tunnel: w520 -> [_ w545]
                    tunnel: [w536 w542] -> w519
                    tunnel: w515 -> [w536 w541]
                    tunnel: w511 -> [_ w540]
                    frame False {
                    }
                    frame True {
                      # "write after interval has passed, else append"
                      n128 = Tick Count (ms)() -> (millisecond timer value=w544:u32)
                      n129 = Subtract(x=w544, y=w541) -> (x-y=w546:u32)
                      n130 = Bundle By Name(cluster=T7 {"Time Stamp"=timestamp(0 s since 1904-01-01), "dt (ms)"=0, "Environmental state values"={"Thermistor (degC)"=0.0, "Sensor temp. (degC)"=0.0, "P_atmos (Pa)"=0.0, "Rel. Humidity (%)"=0.0, "Density (kg/m^3)"=0.0, "Dew point (degC)"=0.0, "Pressure alt. (m)"=0.0, "Density alt. (m)"=0.0}, "Inertial state values"={"w_x (dps)"=0.0, "w_y (dps)"=0.0, "w_z (dps)"=0.0, "a_x (g)"=0.0, "a_y (g)"=0.0, "a_z (g)"=0.0, "Stale sample"=0, "Sensor temp. (degC)"=0.0}} ("All state values"), "Time Stamp"=w554, "dt (ms)"=w540, "Environmental state values"=w556, "Inertial state values"=w555) -> (w549:T7)
                      n131 = Greater Or Equal?(x=w546, y=w545) -> (x >= y?=w543:bool)
                      n132 = case shown="True" w543 {
                        tunnel: [w559 w572] -> w553
                        tunnel: w552 -> [w559 w571]
                        tunnel: w551 -> [w560 w570]
                        tunnel: [w560 w569] -> w550
                        tunnel: w549 -> [w562 w568]
                        tunnel: w547 -> [w563 w567]
                        tunnel: [w561 T7[] []] -> w548
                        tunnel: w544 -> [_ w564]
                        tunnel: [w558 w564] -> w542
                        tunnel: w541 -> [w558 _]
                        frame False {
                          n133 = Build Array (concatenate)(w563, w562) -> (w561:T7[])
                        }
                        frame True {
                          n134 = Build Array (concatenate)(w567, w568) -> (w566:T7[])
                          n135 = call "Datalog append STATE.vi"("Datalog (State) path"=w570, "All state values"=w566, "Error in"=w571) -> ("Path out"=w569:path, "Error out"=w572:errorcluster)  [unwired: 5 in]
                        }
                      }
                    }
                  }
                }
                frame Default {
                }
              }
              "Clock drift" <- w239
              n136 = Or(x="Stop streaming", y=w260) -> (x .or. y?=w259:bool)
            }
            n137 = local read "Data rate (Hz)"() -> (w153:dbl)
            n138 = Reciprocal(x=w153) -> (1/x=w152:dbl)
            n139 = property on="Pressures time trace" class="WFChart (strict)"("XScale.Multiplier"=w152) -> ()  [unwired: 2 in, 2 out]
            n140 = property on="Sensor temperatures time trace (Mode \"P & T\" only)" class="WFChart (strict)"("XScale.Multiplier"=w152) -> ()  [unwired: 2 in, 2 out]
            n141 = call "Stop data stream (s).vi"("VISA resource name in"=w189, "Error In"=w190) -> ("VISA resource name out"=w187:refnum<visa-resource-name>, "Error out"=w188:errorcluster)  [unwired: 7 in]
            n142 = call "Clear buffer.vi"("Error in"=w188, "dt for timeout (ms)"=w185, "VISA resource name in"=w187) -> ("Error out"=w133:errorcluster, "VISA resource name out"=w134:refnum<visa-resource-name>)  [unwired: 3 in]
            n143 = case shown="True" "Save data" {
              tunnel: w143 -> [_ w207]
              tunnel: w142 -> [w198 w206]
              tunnel: w141 -> [_ w205]
              tunnel: w140 -> [_ w204]
              tunnel: w139 -> [_ w203]
              tunnel: w138 -> [_ w202]
              tunnel: [w198 w200] -> w137
              tunnel: w136 -> [_ w199]
              frame False {
              }
              frame True {
                n144 = case shown="0, Default" w204 {
                  tunnel: w207 -> [_ w215]
                  tunnel: w206 -> [w211 w214]
                  tunnel: [w210 w213] -> w201
                  tunnel: w205 -> [w208 w212]
                  tunnel: w203 -> [w209 _]
                  frame 0, Default {
                    n145 = call "Datalog append DATA, Mode 0.vi"("Datalog (Data) path"=w208, "Data (Mode 0)"=w209, "Error in"=w211) -> ("Error out"=w210:errorcluster)  [unwired: 5 in, 1 out]
                  }
                  frame 1 {
                    n146 = call "Datalog append DATA, Mode 1.vi"("Datalog (Data) path"=w212, "Data (Mode 1)"=w215, "Error in"=w214) -> ("Error out"=w213:errorcluster)  [unwired: 5 in, 1 out]
                  }
                }
                n147 = call "Datalog append STATE.vi"("Datalog (State) path"=w199, "All state values"=w202, "Error in"=w201) -> ("Error out"=w200:errorcluster)  [unwired: 5 in, 1 out]
              }
            }
            n148 = call "Close serial port.vi"("Error in"=w133, "VISA resource name"=w134) -> ("Error out"=w184:errorcluster)  [unwired: 9 in]
            n149 = Merge Errors(w184, w137) -> (w183:errorcluster)
          }
        }
        n150 = Dequeue Element(queue=w125, error in (no error)=w124) -> (error out=w123:errorcluster)  [unwired: 1 in, 3 out]
      }
      frame "T" {
        # "dequeue \"busy\" status"
        n151 = Enqueue Element At Opposite End(queue=w600, element=T6 "Busy" ("Cmd"), error in (no error)=w599) -> (queue out=w598:refnum<queue>, error out=w597:errorcluster)  [unwired: 1 in, 1 out]
        n152 = flat-sequence {
          tunnel: w598 -> [w613]
          tunnel: w597 -> [w612]
          tunnel: [w613] -> w596
          tunnel: [w612] -> w595
          tunnel: [TRUE] -> w593
          tunnel: [w606] -> w592
          frame #0 {
            n153 = local read "Serial port"() -> (w605:refnum<visa-resource-name>)
            n154 = Divide(x=1000000.0, y="Data rate (Hz)") -> (x/y=w603:dbl)
            n155 = call "Open serial port.vi"("VISA resource name"=w605) -> ("Error out"=w609:errorcluster, "VISA resource name out"=w610:refnum<visa-resource-name>)  [unwired: 9 in]
            n156 = call "Set stream dt (T).vi"("Error In"=w609, "dt (us)"=w603, "VISA resource name in"=w610) -> ("Error out"=w608:errorcluster, "ACK"=→"ACK 2":bool, "VISA resource name out"=w607:refnum<visa-resource-name>)  [unwired: 6 in]
            n157 = call "Close serial port.vi"("Error in"=w608, "VISA resource name"=w607) -> ("Error out"=w606:errorcluster)  [unwired: 9 in]
          }
        }
        n158 = Dequeue Element(queue=w596, error in (no error)=w595) -> (error out=w594:errorcluster)  [unwired: 1 in, 3 out]
      }
      frame "t" {
        # "dequeue \"busy\" status"
        n159 = Enqueue Element At Opposite End(queue=w625, element=T6 "Busy" ("Cmd"), error in (no error)=w624) -> (queue out=w623:refnum<queue>, error out=w622:errorcluster)  [unwired: 1 in, 1 out]
        n160 = flat-sequence {
          tunnel: w623 -> [w637]
          tunnel: w622 -> [w636]
          tunnel: [w637] -> w621
          tunnel: [w636] -> w620
          tunnel: [TRUE] -> w618
          tunnel: [w630] -> w617
          frame #0 {
            n161 = local read "Env. period (ms)"() -> (w627:i32)
            n162 = local read "Serial port"() -> (w628:refnum<visa-resource-name>)
            n163 = To Unsigned Long Integer(number=w627) -> (unsigned 32bit integer=w626:u32)
            n164 = call "Open serial port.vi"("VISA resource name"=w628) -> ("Error out"=w633:errorcluster, "VISA resource name out"=w634:refnum<visa-resource-name>)  [unwired: 9 in]
            n165 = call "Set state dt (t).vi"("Error In"=w633, "dt (ms)"=w626, "VISA resource name in"=w634) -> ("Error out"=w632:errorcluster, "ACK"=w629:bool, "VISA resource name out"=w631:refnum<visa-resource-name>)  [unwired: 6 in]
            n166 = call "Close serial port.vi"("Error in"=w632, "VISA resource name"=w631) -> ("Error out"=w630:errorcluster)  [unwired: 9 in]
            n167 = local write "ACK 2"(w629) -> ()
          }
        }
        n168 = Dequeue Element(queue=w621, error in (no error)=w620) -> (error out=w619:errorcluster)  [unwired: 1 in, 3 out]
      }
      frame "M" {
        # "dequeue \"busy\" status"
        n169 = Enqueue Element At Opposite End(queue=w649, element=T6 "Busy" ("Cmd"), error in (no error)=w648) -> (queue out=w647:refnum<queue>, error out=w646:errorcluster)  [unwired: 1 in, 1 out]
        n170 = flat-sequence {
          tunnel: w647 -> [w661]
          tunnel: w646 -> [w660]
          tunnel: [w661] -> w645
          tunnel: [w660] -> w644
          tunnel: [TRUE] -> w642
          tunnel: [w654] -> w641
          frame #0 {
            n171 = local read "Serial port"() -> (w652:refnum<visa-resource-name>)
            n172 = call "Open serial port.vi"("VISA resource name"=w652) -> ("Error out"=w657:errorcluster, "VISA resource name out"=w658:refnum<visa-resource-name>)  [unwired: 9 in]
            n173 = call "Set mode (M).vi"("Error In"=w657, "Mode"="Data mode", "VISA resource name in"=w658) -> ("Error out"=w656:errorcluster, "ACK"=w653:bool, "L_data"=→"L_data (bytes)":u16, "VISA resource name out"=w655:refnum<visa-resource-name>)  [unwired: 5 in]
            n174 = call "Close serial port.vi"("Error in"=w656, "VISA resource name"=w655) -> ("Error out"=w654:errorcluster)  [unwired: 9 in]
            n175 = local write "ACK 2"(w653) -> ()
          }
        }
        n176 = Dequeue Element(queue=w645, error in (no error)=w644) -> (error out=w643:errorcluster)  [unwired: 1 in, 3 out]
      }
      frame "O" {
        # "dequeue \"busy\" status"
        n177 = Enqueue Element At Opposite End(queue=w673, element=T6 "Busy" ("Cmd"), error in (no error)=w672) -> (queue out=w671:refnum<queue>, error out=w670:errorcluster)  [unwired: 1 in, 1 out]
        n178 = flat-sequence {
          tunnel: w671 -> [w685]
          tunnel: w670 -> [w684]
          tunnel: [w685] -> w669
          tunnel: [w684] -> w668
          tunnel: [TRUE] -> w666
          tunnel: [w678] -> w665
          frame #0 {
            n179 = local read "Serial port"() -> (w677:refnum<visa-resource-name>)
            n180 = call "Open serial port.vi"("VISA resource name"=w677) -> ("Error out"=w681:errorcluster, "VISA resource name out"=w682:refnum<visa-resource-name>)  [unwired: 9 in]
            n181 = call "Override maxSensorNum (O).vi"("Error In"=w681, "Max. number of sensors"="Max. num. sensors (override)", "VISA resource name in"=w682) -> ("Error out"=w680:errorcluster, "ACK"=→"ACK 3":bool, "L_data"=w674:u16, "VISA resource name out"=w679:refnum<visa-resource-name>)  [unwired: 5 in]
            n182 = local write "L_data (bytes)"(w674) -> ()
            n183 = call "Close serial port.vi"("Error in"=w680, "VISA resource name"=w679) -> ("Error out"=w678:errorcluster)  [unwired: 9 in]
          }
        }
        n184 = Dequeue Element(queue=w669, error in (no error)=w668) -> (error out=w667:errorcluster)  [unwired: 1 in, 3 out]
      }
      frame "G" {
        # "dequeue \"busy\" status"
        n185 = Enqueue Element At Opposite End(queue=w697, element=T6 "Busy" ("Cmd"), error in (no error)=w696) -> (queue out=w695:refnum<queue>, error out=w694:errorcluster)  [unwired: 1 in, 1 out]
        n186 = flat-sequence {
          tunnel: w695 -> [w713]
          tunnel: w694 -> [w712]
          tunnel: [w713] -> w693
          tunnel: [w712] -> w692
          tunnel: [TRUE] -> w690
          tunnel: [w706] -> w689
          frame #0 {
            n187 = local read "Serial port"() -> (w705:refnum<visa-resource-name>)
            n188 = call "Open serial port.vi"("VISA resource name"=w705) -> ("Error out"=w709:errorcluster, "VISA resource name out"=w710:refnum<visa-resource-name>)  [unwired: 9 in]
            n189 = call "Get status bits 1 (G).vi"("VISA resource name in"=w710, "Error In"=w709) -> ("nFaults"=w702:u8, "nSensors"=w701:u8, "nCards"=w700:u8, "PowerState"=w699:bool, "VISA resource name out"=w707:refnum<visa-resource-name>, "ACK"=→"ACK 5":bool, "Error out"=w708:errorcluster)  [unwired: 11 in]
            n190 = local read "System status"() -> (w698:T4)
            n191 = call "Close serial port.vi"("Error in"=w708, "VISA resource name"=w707) -> ("Error out"=w706:errorcluster)  [unwired: 9 in]
            n192 = Bundle By Name(cluster=w698, "Main power"=w699, "Occupied slots"=w700, "Active sensors"=w701, "Faulty sensors"=w702) -> (→"System status":T4)
          }
        }
        n193 = Dequeue Element(queue=w693, error in (no error)=w692) -> (error out=w691:errorcluster)  [unwired: 1 in, 3 out]
      }
      frame "g" {
        # "dequeue \"busy\" status"
        n194 = Enqueue Element At Opposite End(queue=w725, element=T6 "Busy" ("Cmd"), error in (no error)=w724) -> (queue out=w723:refnum<queue>, error out=w722:errorcluster)  [unwired: 1 in, 1 out]
        n195 = flat-sequence {
          tunnel: w723 -> [w746]
          tunnel: w722 -> [w745]
          tunnel: [w746] -> w721
          tunnel: [w745] -> w720
          tunnel: [TRUE] -> w718
          tunnel: [w739] -> w717
          frame #0 {
            w728 = T10."Disabled and Grayed Out" ("Disabled")
            w727 = T10."Enabled" ("Disabled")
            n196 = local read "Serial port"() -> (w738:refnum<visa-resource-name>)
            n197 = call "Open serial port.vi"("VISA resource name"=w738) -> ("Error out"=w742:errorcluster, "VISA resource name out"=w743:refnum<visa-resource-name>)  [unwired: 9 in]
            n198 = call "Get status bits 2 (g).vi"("VISA resource name in"=w743, "Error In"=w742) -> ("Mode"=w737:u8, "Therm_ok"=w729:bool, "BMI160_ok"=w733:bool, "BME280_ok"=w731:bool, "VISA resource name out"=w740:refnum<visa-resource-name>, "ACK"=w735:bool, "Error out"=w741:errorcluster)  [unwired: 11 in]
            n199 = Select(t=w727, s=w729, f=w728) -> (s? t:f=w732:T10)
            n200 = Select(t=w727, s=w731, f=w728) -> (s? t:f=w730:T10)
            n201 = stacked-sequence {
              tunnel: w732 -> [_ w748]
              tunnel: w730 -> [w747 _]
              tunnel: w729 -> [_ w749]
              frame #0 {
                n202 = property on="Environmental state values" class="Clust (strict)"("DisabledEnum"=w747) -> ()  [unwired: 2 in, 2 out]
                n203 = property on="Density (kg/m^3)" class="DigNum (strict)"("DisabledEnum"=w747) -> ()  [unwired: 2 in, 2 out]
                n204 = property on="Dew point (degC)" class="DigNum (strict)"("DisabledEnum"=w747) -> ()  [unwired: 2 in, 2 out]
                n205 = property on="Density alt. (m)" class="DigNum (strict)"("DisabledEnum"=w747) -> ()  [unwired: 2 in, 2 out]
              }
              frame #1 {
                n206 = case shown="False" w749 {
                  tunnel: w748 -> [w750 _]
                  frame False {
                    n207 = property on="Density (kg/m^3)" class="DigNum (strict)"("DisabledEnum"=w750) -> ()  [unwired: 2 in, 2 out]
                    n208 = property on="Dew point (degC)" class="DigNum (strict)"("DisabledEnum"=w750) -> ()  [unwired: 2 in, 2 out]
                    n209 = property on="Density alt. (m)" class="DigNum (strict)"("DisabledEnum"=w750) -> ()  [unwired: 2 in, 2 out]
                  }
                  frame True {
                  }
                }
                n210 = property on="Thermistor (degC)" class="DigNum (strict)"("DisabledEnum"=w748) -> ()  [unwired: 2 in, 2 out]
              }
            }
            n211 = local read "System status"() -> (w734:T4)
            n212 = call "Close serial port.vi"("Error in"=w741, "VISA resource name"=w740) -> ("Error out"=w739:errorcluster)  [unwired: 9 in]
            n213 = local write "ACK 5"(w735) -> ()
            n214 = Select(t=w727, s=w733, f=w728) -> (s? t:f=w726:T10)
            n215 = Bundle By Name(cluster=w734, "Env. sensor"=w731, "Inertial sensor"=w733, "Thermistor"=w729, "Mode"=w737) -> (w736:T4)
            n216 = property on="Inertial state values" class="Clust (strict)"("DisabledEnum"=w726) -> ()  [unwired: 2 in, 2 out]
            n217 = property on="AccelGyro constants" class="Clust (strict)"("DisabledEnum"=w726) -> ()  [unwired: 2 in, 2 out]
            n218 = property on="Accel. range (g)" class="Ring (strict)"("DisabledEnum"=w726) -> ()  [unwired: 2 in, 2 out]
            n219 = property on="Accel. rate (Hz)" class="Ring (strict)"("DisabledEnum"=w726) -> ()  [unwired: 2 in, 2 out]
            n220 = property on="Gyro. range (dps)" class="Ring (strict)"("DisabledEnum"=w726) -> ()  [unwired: 2 in, 2 out]
            n221 = property on="Gyro. rate (Hz)" class="Ring (strict)"("DisabledEnum"=w726) -> ()  [unwired: 2 in, 2 out]
            n222 = property on="Apply settings 3" class="Bool"("DisabledEnum"=w726) -> ()  [unwired: 2 in, 2 out]
            n223 = property on="ACK 8" class="Bool (strict)"("DisabledEnum"=w726) -> ()  [unwired: 2 in, 2 out]
            n224 = local write "System status"(w736) -> ()
          }
        }
        n225 = Dequeue Element(queue=w721, error in (no error)=w720) -> (error out=w719:errorcluster)  [unwired: 1 in, 3 out]
      }
      frame "F" {
        # "dequeue \"busy\" status"
        n226 = Enqueue Element At Opposite End(queue=w762, element=T6 "Busy" ("Cmd"), error in (no error)=w761) -> (queue out=w760:refnum<queue>, error out=w759:errorcluster)  [unwired: 1 in, 1 out]
        n227 = flat-sequence {
          tunnel: w760 -> [w772]
          tunnel: w759 -> [w771]
          tunnel: [w772] -> w758
          tunnel: [w771] -> w757
          tunnel: [TRUE] -> w755
          tunnel: [w765] -> w754
          frame #0 {
            n228 = local read "Serial port"() -> (w764:refnum<visa-resource-name>)
            n229 = call "Open serial port.vi"("VISA resource name"=w764) -> ("Error out"=w768:errorcluster, "VISA resource name out"=w769:refnum<visa-resource-name>)  [unwired: 9 in]
            n230 = call "Collate faulty sensor indices.vi"("Error In"=w768, "VISA resource name in"=w769) -> ("Error out"=w767:errorcluster, "Faulty sensor indices"=→"Faulty sensors":i32[], "VISA resource name out"=w766:refnum<visa-resource-name>)  [unwired: 7 in]
            n231 = call "Close serial port.vi"("Error in"=w767, "VISA resource name"=w766) -> ("Error out"=w765:errorcluster)  [unwired: 9 in]
          }
        }
        n232 = Dequeue Element(queue=w758, error in (no error)=w757) -> (error out=w756:errorcluster)  [unwired: 1 in, 3 out]
      }
      frame "A" {
        # "dequeue \"busy\" status"
        n233 = Enqueue Element At Opposite End(queue=w784, element=T6 "Busy" ("Cmd"), error in (no error)=w783) -> (queue out=w782:refnum<queue>, error out=w781:errorcluster)  [unwired: 1 in, 1 out]
        n234 = flat-sequence {
          tunnel: w782 -> [w794]
          tunnel: w781 -> [w793]
          tunnel: [w794] -> w780
          tunnel: [w793] -> w779
          tunnel: [TRUE] -> w777
          tunnel: [w787] -> w776
          frame #0 {
            n235 = local read "Serial port"() -> (w786:refnum<visa-resource-name>)
            n236 = call "Open serial port.vi"("VISA resource name"=w786) -> ("Error out"=w790:errorcluster, "VISA resource name out"=w791:refnum<visa-resource-name>)  [unwired: 9 in]
            n237 = call "Collate active sensor indices.vi"("Error In"=w790, "VISA resource name in"=w791) -> ("Error out"=w789:errorcluster, "Active sensor indices"=→"Active sensors":i32[], "VISA resource name out"=w788:refnum<visa-resource-name>)  [unwired: 7 in]
            n238 = call "Close serial port.vi"("Error in"=w789, "VISA resource name"=w788) -> ("Error out"=w787:errorcluster)  [unwired: 9 in]
          }
        }
        n239 = Dequeue Element(queue=w780, error in (no error)=w779) -> (error out=w778:errorcluster)  [unwired: 1 in, 3 out]
      }
      frame "C" {
        # "dequeue \"busy\" status"
        n240 = Enqueue Element At Opposite End(queue=w806, element=T6 "Busy" ("Cmd"), error in (no error)=w805) -> (queue out=w804:refnum<queue>, error out=w803:errorcluster)  [unwired: 1 in, 1 out]
        n241 = flat-sequence {
          tunnel: w804 -> [w824]
          tunnel: w803 -> [w823]
          tunnel: [w824] -> w802
          tunnel: [w823] -> w801
          tunnel: [TRUE] -> w799
          tunnel: [w817] -> w798
          frame #0 {
            n242 = local read "Serial port"() -> (w816:refnum<visa-resource-name>)
            n243 = call "Open serial port.vi"("VISA resource name"=w816) -> ("Error out"=w820:errorcluster, "VISA resource name out"=w821:refnum<visa-resource-name>)  [unwired: 9 in]
            n244 = call "Configure BMI160 (C).vi"("VISA resource name in"=w821, "Accel. range (g)"="Accel. range (g)", "Accel. rate (Hz)"="Accel. rate (Hz)", "Gyro. range (dps)"="Gyro. range (dps)", "Gyro. rate (Hz)"="Gyro. rate (Hz)", "Error In"=w820) -> ("VISA resource name out"=w818:refnum<visa-resource-name>, "ACK ok"=→"ACK 4":bool, "Error out"=w819:errorcluster)  [unwired: 11 in]
            n245 = case shown="0, Default" "Accel. range (g)" {
              tunnel: [sgl 2.0 ("accRange") sgl 4.0 ("accRange") sgl 8.0 ("accRange") sgl 16.0 ("accRange")] -> w810
              frame 0, Default {
              }
              frame 1 {
              }
              frame 2 {
              }
              frame 3 {
              }
            }
            n246 = case shown="0, Default" "Gyro. range (dps)" {
              tunnel: [sgl 125.0 ("accRange") sgl 250.0 ("accRange") sgl 500.0 ("accRange") sgl 1000.0 ("accRange") sgl 2000.0 ("accRange")] -> w808
              frame 0, Default {
              }
              frame 1 {
              }
              frame 2 {
              }
              frame 3 {
              }
              frame 4 {
              }
            }
            n247 = call "Close serial port.vi"("Error in"=w819, "VISA resource name"=w818) -> ("Error out"=w817:errorcluster)  [unwired: 9 in]
            n248 = local read "AccelGyro constants"() -> (w807:T1)
            n249 = Bundle By Name(cluster=w807, "accRange"=w810, "gyrRange"=w808) -> (w812:T1)
            n250 = local write "AccelGyro constants"(w812) -> ()
          }
        }
        n251 = Dequeue Element(queue=w802, error in (no error)=w801) -> (error out=w800:errorcluster)  [unwired: 1 in, 3 out]
      }
      frame "Z" {
        # "dequeue \"busy\" status"
        n252 = Enqueue Element At Opposite End(queue=w845, element=T6 "Busy" ("Cmd"), error in (no error)=w844) -> (queue out=w843:refnum<queue>, error out=w842:errorcluster)  [unwired: 1 in, 1 out]
        n253 = flat-sequence {
          tunnel: w843 -> [w855]
          tunnel: w842 -> [w854]
          tunnel: [w855] -> w841
          tunnel: [w854] -> w840
          tunnel: [TRUE] -> w838
          tunnel: [w848] -> w837
          frame #0 {
            n254 = local read "Serial port"() -> (w847:refnum<visa-resource-name>)
            n255 = call "Open serial port.vi"("VISA resource name"=w847) -> ("Error out"=w851:errorcluster, "VISA resource name out"=w852:refnum<visa-resource-name>)  [unwired: 9 in]
            n256 = call "Get Serial Number (Z).vi"("VISA resource name in"=w852, "Error In"=w851) -> ("VISA resource name out"=w849:refnum<visa-resource-name>, "Serial Number"=→"Serial no.":u16, "Error out"=w850:errorcluster)  [unwired: 5 in, 1 out]
            n257 = call "Close serial port.vi"("Error in"=w850, "VISA resource name"=w849) -> ("Error out"=w848:errorcluster)  [unwired: 9 in]
          }
        }
        n258 = Dequeue Element(queue=w841, error in (no error)=w840) -> (error out=w839:errorcluster)  [unwired: 1 in, 3 out]
      }
      frame "D" {
        # "dequeue \"busy\" status"
        n259 = Enqueue Element At Opposite End(queue=w869, element=T6 "Busy" ("Cmd"), error in (no error)=w868) -> (queue out=w867:refnum<queue>, error out=w866:errorcluster)  [unwired: 1 in, 1 out]
        n260 = flat-sequence {
          tunnel: w867 -> [w892]
          tunnel: w866 -> [w891]
          tunnel: [w892] -> w865
          tunnel: [w891] -> w864
          tunnel: [TRUE] -> w862
          tunnel: [w873] -> w861
          tunnel: [w871] -> w859
          tunnel: w858 -> [w877]
          tunnel: w857 -> [w876]
          tunnel: [w875] -> w856
          frame #0 {
            n261 = local read "Save data"() -> (w872:bool)
            n262 = local read "AccelGyro constants"() -> (w881:T1)
            n263 = local read "Serial port"() -> (w889:refnum<visa-resource-name>)
            n264 = call "Open serial port.vi"("VISA resource name"=w889) -> ("Error out"=w887:errorcluster, "VISA resource name out"=w888:refnum<visa-resource-name>)  [unwired: 9 in]
            n265 = call "Get Env data (oneshot) (D).vi"("VISA resource name in"=w888, "Error In"=w887) -> ("VISA resource name out"=w885:refnum<visa-resource-name>, "STATE_Buffer"=w884:string, "ACK"=→"ACK 6":bool, "Error out"=w886:errorcluster)  [unwired: 5 in]
            n266 = call "Close serial port.vi"("Error in"=w886, "VISA resource name"=w885) -> ("Error out"=w874:errorcluster)  [unwired: 9 in]
            n267 = String Subset(string=w884, offset (0)=1) -> (substring=w883:string)  [unwired: 1 in]
            n268 = call "Process State Buffer.vi"("AccelGyro constants"=w881, "STATE_Buffer excluding '$' [1...30]"=w883) -> ("Inertial state values"=w878:T2, "Environmental state values"=w879:T3)
            n269 = case shown="True" w872 {
              tunnel: w879 -> [_ w916]
              tunnel: w878 -> [_ w915]
              tunnel: [errorcluster {"status"=FALSE, "code"=0, "source"=""} ("Error out") w913] -> w870
              tunnel: [w895 w911] -> w871
              tunnel: w877 -> [w895 w910]
              tunnel: w876 -> [w894 w905]
              tunnel: [w894 w906] -> w875
              frame False {
                (unwired) path "" ("Path out")
              }
              frame True {
                # "write after interval has passed, else append"
                n270 = local read "Datalog name (without extension)"() -> (w898:string)
                n271 = local read "Datalog directory"() -> (w899:path)
                n272 = local read "Write interval (s)"() -> (w903:u32)
                n273 = Concatenate Strings(w898, "_S_.log" ("string")) -> (w900:string)
                n274 = local read "Env. period (ms)"() -> (w914:i32)
                n275 = Get Date/Time In Seconds() -> (seconds since 1Jan1904=w904:timestamp)
                n276 = Build Path(base path=w899, name or relative path=w900) -> (appended path=w897:path)
                n277 = Multiply(x=u32 1000, y=w903) -> (x*y=w902:u32)
                n278 = Tick Count (ms)() -> (millisecond timer value=w908:u32)
                n279 = Subtract(x=w908, y=w905) -> (x-y=w909:u32)
                n280 = Bundle By Name(cluster=T7 {"Time Stamp"=timestamp(0 s since 1904-01-01), "dt (ms)"=0, "Environmental state values"={"Thermistor (degC)"=0.0, "Sensor temp. (degC)"=0.0, "P_atmos (Pa)"=0.0, "Rel. Humidity (%)"=0.0, "Density (kg/m^3)"=0.0, "Dew point (degC)"=0.0, "Pressure alt. (m)"=0.0, "Density alt. (m)"=0.0}, "Inertial state values"={"w_x (dps)"=0.0, "w_y (dps)"=0.0, "w_z (dps)"=0.0, "a_x (g)"=0.0, "a_y (g)"=0.0, "a_z (g)"=0.0, "Stale sample"=0, "Sensor temp. (degC)"=0.0}} ("All state values"), "Time Stamp"=w904, "dt (ms)"=w914, "Environmental state values"=w916, "Inertial state values"=w915) -> (w912:T7)
                n281 = Greater Or Equal?(x=w909, y=w902) -> (x >= y?=w907:bool)
                n282 = case shown="True" w907 {
                  tunnel: [errorcluster {"status"=FALSE, "code"=0, "source"=""} ("Error out") w930] -> w913
                  tunnel: w897 -> [_ w929]
                  tunnel: w912 -> [w921 w928]
                  tunnel: w910 -> [w922 w927]
                  tunnel: [w920 T7[] []] -> w911
                  tunnel: w908 -> [_ w924]
                  tunnel: [w919 w924] -> w906
                  tunnel: w905 -> [w919 _]
                  frame False {
                    n283 = Build Array (concatenate)(w922, w921) -> (w920:T7[])
                  }
                  frame True {
                    n284 = Build Array (concatenate)(w927, w928) -> (w926:T7[])
                    n285 = call "Datalog append STATE.vi"("Datalog (State) path"=w929, "All state values"=w926, "Error in"=errorcluster {"status"=FALSE, "code"=0, "source"=""} ("Error out")) -> ("Error out"=w930:errorcluster)  [unwired: 5 in, 1 out]
                  }
                }
              }
            }
            n286 = local write "Environmental state values"(w879) -> ()
            n287 = local write "Inertial state values"(w878) -> ()
            n288 = Merge Errors(w874, w870) -> (w873:errorcluster)
          }
        }
        n289 = Dequeue Element(queue=w865, error in (no error)=w864) -> (error out=w863:errorcluster)  [unwired: 1 in, 3 out]
      }
      frame "accgyr_consts" {
        # "dequeue \"busy\" status"
        n290 = Enqueue Element At Opposite End(queue=w942, element=T6 "Busy" ("Cmd"), error in (no error)=w941) -> (queue out=w940:refnum<queue>, error out=w939:errorcluster)  [unwired: 1 in, 1 out]
        n291 = flat-sequence {
          tunnel: w940 -> [w962]
          tunnel: w939 -> [w961]
          tunnel: [w962] -> w938
          tunnel: [w961] -> w937
          tunnel: [TRUE] -> w935
          tunnel: [w959] -> w934
          frame #0 {
            n292 = local read "Serial port"() -> (w958:refnum<visa-resource-name>)
            n293 = call "Open serial port.vi"("VISA resource name"=w958) -> ("Error out"=w956:errorcluster, "VISA resource name out"=w957:refnum<visa-resource-name>)  [unwired: 9 in]
            n294 = call "Get AccelGyro constants (MCU EEPROM).vi"("VISA resource name in"=w957, "Error In"=w956) -> ("VISA resource name out"=w954:refnum<visa-resource-name>, "AccelGyro constants"=w951:T1, "ACK"=→"ACK 8":bool, "Error out"=w955:errorcluster)  [unwired: 5 in]
            n295 = Unbundle By Name(w951) -> ("gx offset"=w950:sgl, "gy offset"=w949:sgl, "gz offset"=w948:sgl, "ax offset"=w947:sgl, "ay offset"=w946:sgl, "az offset"=w945:sgl, "axyz scale"=w944:sgl)
            n296 = call "Close serial port.vi"("Error in"=w955, "VISA resource name"=w954) -> ("Error out"=w959:errorcluster)  [unwired: 9 in]
            n297 = Bundle By Name(cluster=T1 {"gyrRange"=125.0, "accRange"=2.0, "gx offset"=0.0, "gy offset"=0.0, "gz offset"=0.0, "ax offset"=0.0, "ay offset"=0.0, "az offset"=0.0, "axyz scale"=1.0} ("AccelGyro constants"), "gx offset"=w950, "gy offset"=w949, "gz offset"=w948, "ax offset"=w947, "ay offset"=w946, "az offset"=w945, "axyz scale"=w944) -> (→"AccelGyro constants":T1)
          }
        }
        n298 = Dequeue Element(queue=w938, error in (no error)=w937) -> (error out=w936:errorcluster)  [unwired: 1 in, 3 out]
      }
      frame "EEPROM_Pconsts" {
        # "dequeue \"busy\" status"
        n299 = Enqueue Element At Opposite End(queue=w974, element=T6 "Busy" ("Cmd"), error in (no error)=w973) -> (queue out=w972:refnum<queue>, error out=w971:errorcluster)  [unwired: 1 in, 1 out]
        n300 = flat-sequence {
          tunnel: w972 -> [w990]
          tunnel: w971 -> [w989]
          tunnel: [w990] -> w970
          tunnel: [w989] -> w969
          tunnel: [TRUE] -> w967
          tunnel: [w987] -> w966
          frame #0 {
            # "Must only run this case after running \"P\", \"G\", \"A\""
            n301 = local read "System status"() -> (w979:T4)
            n302 = Unbundle By Name(w979) -> ("Occupied slots"=w978:u8)
            n303 = local read "Serial port"() -> (w986:refnum<visa-resource-name>)
            n304 = To Long Integer(number=w978) -> (32bit integer=w977:i32)
            n305 = call "Open serial port.vi"("VISA resource name"=w986) -> ("Error out"=w984:errorcluster, "VISA resource name out"=w985:refnum<visa-resource-name>)  [unwired: 9 in]
            n306 = local read "Active sensors"() -> (w981:i32[])
            n307 = call "Concatenate all slot EEPROM arrays.vi"("Error In"=w984, "N slots occupied"=w977, "VISA resource name in"=w985) -> ("Error out"=w983:errorcluster, "ACK (all)"=→"ACK 7":bool, "All slot EEPROM values"=w976:T11[], "VISA resource name out"=w982:refnum<visa-resource-name>)  [unwired: 5 in]
            n308 = call "Populate pressure constants array.vi"("Occupied slot EEPROM values"=w976, "Active sensor indices"=w981) -> ("Active pressure sensor constants"=→"Active pressure sensor constants":T5[])
            n309 = call "Close serial port.vi"("Error in"=w983, "VISA resource name"=w982) -> ("Error out"=w987:errorcluster)  [unwired: 9 in]
          }
        }
        n310 = Dequeue Element(queue=w970, error in (no error)=w969) -> (error out=w968:errorcluster)  [unwired: 1 in, 3 out]
      }
      frame "convert_datalogs" {
        # "dequeue \"busy\" status"
        n311 = Enqueue Element At Opposite End(queue=w1002, element=T6 "Busy" ("Cmd"), error in (no error)=w1001) -> (queue out=w1000:refnum<queue>, error out=w999:errorcluster)  [unwired: 1 in, 1 out]
        n312 = flat-sequence {
          tunnel: w1000 -> [w1052]
          tunnel: w999 -> [w1051]
          tunnel: [w1052] -> w998
          tunnel: [w1051] -> w997
          tunnel: [TRUE] -> w995
          tunnel: [w1031] -> w994
          frame #0 {
            n313 = local read "System status"() -> (w1042:T4)
            n314 = local read "Datalog name (without extension)"() -> (w1039:string)
            n315 = local read "Datalog name (without extension)"() -> (w1046:string)
            n316 = Unbundle By Name(w1042) -> ("Mode"=w1038:u8)
            n317 = local read "Datalog directory"() -> (w1040:path)
            n318 = local read "Datalog directory"() -> (w1047:path)
            n319 = case shown="0, Default" w1038 {
              tunnel: ["_P0.log" ("string") "_P1.log" ("string")] -> w1041
              frame 0, Default {
              }
              frame 1 {
              }
            }
            n320 = Concatenate Strings(w1039, "_S.log" ("string")) -> (w1043:string)
            n321 = Concatenate Strings(w1046, "_S_.log" ("string")) -> (w1048:string)
            n322 = Concatenate Strings(w1039, w1041) -> (w1045:string)
            n323 = Build Path(base path=w1040, name or relative path=w1045) -> (appended path=w1007:path)
            n324 = Build Path(base path=w1040, name or relative path=w1043) -> (appended path=w1015:path)
            n325 = Build Path(base path=w1047, name or relative path=w1048) -> (appended path=w1029:path)
            n326 = Path To String(path=w1015) -> (string=w1016:string)
            n327 = Path To String(path=w1029) -> (string=w1028:string)
            n328 = Path To String(path=w1007) -> (string=w1013:string)
            n329 = Reverse String(1:w1016) -> (0:w1017:string)
            n330 = Reverse String(1:w1028) -> (0:w1027:string)
            n331 = Reverse String(1:w1013) -> (0:w1012:string)
            n332 = String Subset(string=w1017, offset (0)=3 ("length (rest)")) -> (substring=w1018:string)  [unwired: 1 in]
            n333 = String Subset(string=w1027, offset (0)=3 ("length (rest)")) -> (substring=w1026:string)  [unwired: 1 in]
            n334 = String Subset(string=w1012, offset (0)=3 ("length (rest)")) -> (substring=w1011:string)  [unwired: 1 in]
            n335 = Reverse String(1:w1018) -> (0:w1019:string)
            n336 = Reverse String(1:w1026) -> (0:w1025:string)
            n337 = Reverse String(1:w1011) -> (0:w1010:string)
            n338 = Concatenate Strings(w1019, "txt" ("string")) -> (w1021:string)
            n339 = Concatenate Strings(w1025, "txt" ("string")) -> (w1023:string)
            n340 = Concatenate Strings(w1010, "txt" ("string")) -> (w1008:string)
            n341 = String To Path(string=w1021) -> (path=w1014:path)
            n342 = String To Path(string=w1023) -> (path=w1022:path)
            n343 = String To Path(string=w1008) -> (path=w1006:path)
            n344 = case shown="0, Default" w1038 {
              tunnel: w1007 -> [w1059 w1063]
              tunnel: [w1057 w1061] -> w1034
              tunnel: "d.p" -> [w1056 w1064]
              tunnel: w1006 -> [w1055 w1060]
              frame 0, Default {
                n345 = call "Datalog to ASCII (DATA, Mode 0).vi"("Error in"=errorcluster {"status"=FALSE, "code"=0, "source"=""}, "ASCII output path"=w1055, "Precision"=w1056, "Datalog path"=w1059) -> ("Error out"=w1057:errorcluster)  [unwired: 3 in]
              }
              frame 1 {
                n346 = call "Datalog to ASCII (DATA, Mode 1).vi"("Error in"=errorcluster {"status"=FALSE, "code"=0, "source"=""}, "ASCII output path"=w1060, "Precision"=w1064, "Datalog path"=w1063) -> ("Error out"=w1061:errorcluster)  [unwired: 3 in]
              }
            }
            n347 = call "Datalog to ASCII (STATE).vi"("Error in"=errorcluster {"status"=FALSE, "code"=0, "source"=""}, "ASCII output path"=w1014, "Precision"="d.p", "Datalog path"=w1015) -> ("Error out"=w1033:errorcluster)  [unwired: 3 in]
            n348 = call "Datalog to ASCII (STATE_).vi"("Error in"=errorcluster {"status"=FALSE, "code"=0, "source"=""}, "ASCII output path"=w1022, "Precision"="d.p", "Datalog path"=w1029) -> ("Error out"=w1032:errorcluster)  [unwired: 3 in]
            n349 = Merge Errors(w1034, w1033, w1032) -> (w1031:errorcluster)
            n350 = case shown="No Error" w1031 {
              tunnel: [TRUE FALSE] -> w1030
              frame No Error {
              }
              frame Error {
              }
            }
            "ASCII done" <- w1030
          }
        }
        n351 = Dequeue Element(queue=w998, error in (no error)=w997) -> (error out=w996:errorcluster)  [unwired: 1 in, 3 out]
      }
      frame "Exit", Default {
      }
    }
    n352 = call <vilib>:"Clear Errors.vi"("error in (no error)"=w39, "specific error code to clear (0: all)"=1073676294) -> ("error out"=w38:errorcluster)  [unwired: 4 in, 1 out]
    "Error" <- w38
  }
  n353 = while {
    tunnel: w10 -> [w1076]
    tunnel: w9 -> [w1075]
    tunnel: [w1074] -> w32
    tunnel: [w1073] -> w31
    stop <- w1077 continue-if-true
    n354 = event shown="[0] Timeout" {
      selector: _ -> [_ _ _ _ _ _ _ _ _ _]
      dyn-events: _ -> [_ _ _ _ _ _ _ _ _ _]
      timeout: "Env. period (ms)" -> [_ _ _ _ _ _ _ _ _ _]
      tunnel: [TRUE TRUE w1169 TRUE TRUE TRUE TRUE TRUE TRUE TRUE] -> w1077
      tunnel: w1076 -> [w1090 w1108 w1173 w1201 w1256 w1274 w1302 w1336 w1358 w1377]
      tunnel: w1075 -> [w1089 w1107 w1174 w1200 w1253 w1273 w1301 w1335 w1357 w1376]
      tunnel: [w1087 w1103 w1178 w1199 w1254 w1271 w1300 w1333 w1356 w1374] -> w1074
      tunnel: [w1088 w1104 w1179 w1198 w1255 w1270 w1299 w1334 w1355 w1375] -> w1073
      event Timeout {
        # "only queue msg if not busy"
        n355 = event-data() -> ()  [unwired: 1 in, 1 out]
        n356 = local read "System status"() -> (w1081:T4)
        n357 = Unbundle By Name(w1081) -> ("Main power"=w1080:bool)
        n358 = Preview Queue Element(queue=w1090, timeout in ms (-1)=0, error in (no error)=w1089) -> (queue out=w1084:refnum<queue>, element=w1086:T6, error out=w1083:errorcluster)  [unwired: 1 out]
        n359 = Not Equal?(x=T6 "Busy" ("Cmd"), y=w1086) -> (x != y?=w1079:bool)
        n360 = And(x=w1080, y=w1079) -> (x .and. y?=w1078:bool)
        n361 = case shown="True" w1078 {
          tunnel: w1084 -> [w1093 w1098]
          tunnel: w1083 -> [w1092 w1097]
          tunnel: [w1093 w1095] -> w1088
          tunnel: [w1092 w1096] -> w1087
          frame False {
          }
          frame True {
            n362 = local write "ACK 6"(FALSE ("ACK 6")) -> ()
            n363 = Enqueue Element(queue=w1098, element=T6 "D" ("Cmd"), error in (no error)=w1097) -> (queue out=w1095:refnum<queue>, error out=w1096:errorcluster)  [unwired: 1 in, 1 out]
          }
        }
      }
      event "Main Power": Value Change {
        # "only queue msg if not busy"
        n364 = event-data() -> ("NewVal"=w1100:bool)  [unwired: 1 in, 1 out]
        n365 = Preview Queue Element(queue=w1108, timeout in ms (-1)=0, error in (no error)=w1107) -> (queue out=w1106:refnum<queue>, element=w1111:T6, error out=w1105:errorcluster)  [unwired: 1 out]
        n366 = Not Equal?(x=T6 "Busy" ("Cmd"), y=w1111) -> (x != y?=w1109:bool)
        n367 = case shown="True" w1109 {
          tunnel: w1106 -> [w1113 w1121]
          tunnel: w1105 -> [w1112 w1122]
          tunnel: [w1113 w1120] -> w1104
          tunnel: [w1112 w1123] -> w1103
          tunnel: w1100 -> [_ w1124]
          frame False {
          }
          frame True {
            n368 = case shown="True" w1124 {
              tunnel: [w1128 w1139] -> w1123
              tunnel: w1122 -> [w1135 w1166]
              tunnel: w1121 -> [w1136 w1167]
              tunnel: [w1127 w1138] -> w1120
              frame False {
                n369 = Enqueue Element(queue=w1136, element=T6 "p" ("Cmd"), error in (no error)=w1135) -> (queue out=w1132:refnum<queue>, error out=w1131:errorcluster)  [unwired: 1 in, 1 out]
                n370 = Enqueue Element(queue=w1132, element=T6 "G" ("Cmd"), error in (no error)=w1131) -> (queue out=w1130:refnum<queue>, error out=w1129:errorcluster)  [unwired: 1 in, 1 out]
                n371 = Enqueue Element(queue=w1130, element=T6 "g" ("Cmd"), error in (no error)=w1129) -> (queue out=w1127:refnum<queue>, error out=w1128:errorcluster)  [unwired: 1 in, 1 out]
              }
              frame True {
                n372 = Enqueue Element(queue=w1167, element=T6 "P" ("Cmd"), error in (no error)=w1166) -> (queue out=w1160:refnum<queue>, error out=w1159:errorcluster)  [unwired: 1 in, 1 out]
                n373 = Enqueue Element(queue=w1160, element=T6 "F" ("Cmd"), error in (no error)=w1159) -> (queue out=w1164:refnum<queue>, error out=w1165:errorcluster)  [unwired: 1 in, 1 out]
                n374 = Enqueue Element(queue=w1164, element=T6 "A" ("Cmd"), error in (no error)=w1165) -> (queue out=w1145:refnum<queue>, error out=w1144:errorcluster)  [unwired: 1 in, 1 out]
                n375 = Enqueue Element(queue=w1145, element=T6 "T" ("Cmd"), error in (no error)=w1144) -> (queue out=w1147:refnum<queue>, error out=w1146:errorcluster)  [unwired: 1 in, 1 out]
                n376 = Enqueue Element(queue=w1147, element=T6 "t" ("Cmd"), error in (no error)=w1146) -> (queue out=w1142:refnum<queue>, error out=w1143:errorcluster)  [unwired: 1 in, 1 out]
                n377 = Enqueue Element(queue=w1142, element=T6 "M" ("Cmd"), error in (no error)=w1143) -> (queue out=w1156:refnum<queue>, error out=w1155:errorcluster)  [unwired: 1 in, 1 out]
                n378 = Enqueue Element(queue=w1156, element=T6 "G" ("Cmd"), error in (no error)=w1155) -> (queue out=w1157:refnum<queue>, error out=w1158:errorcluster)  [unwired: 1 in, 1 out]
                n379 = Enqueue Element(queue=w1157, element=T6 "g" ("Cmd"), error in (no error)=w1158) -> (queue out=w1152:refnum<queue>, error out=w1151:errorcluster)  [unwired: 1 in, 1 out]
                n380 = Enqueue Element(queue=w1152, element=T6 "EEPROM_Pconsts" ("Cmd"), error in (no error)=w1151) -> (queue out=w1141:refnum<queue>, error out=w1140:errorcluster)  [unwired: 1 in, 1 out]
                n381 = Enqueue Element(queue=w1141, element=T6 "C" ("Cmd"), error in (no error)=w1140) -> (queue out=w1138:refnum<queue>, error out=w1139:errorcluster)  [unwired: 1 in, 1 out]
              }
            }
            n382 = local write "ACK 1"(FALSE ("ACK 1")) -> ()
            n383 = local write "ACK 5"(FALSE ("ACK 8")) -> ()
            n384 = local write "ACK 2"(FALSE ("ACK 6")) -> ()
            n385 = local write "ACK 6"(FALSE ("ACK 6")) -> ()
            n386 = local write "ACK 3"(FALSE ("ACK 8")) -> ()
            n387 = local write "ACK 7"(FALSE ("ACK 6")) -> ()
            n388 = local write "ACK 4"(FALSE ("Done")) -> ()
          }
        }
      }
      event "Stop UI": Value Change {
        # "only queue msg if not busy"
        n389 = event-data() -> ()  [unwired: 1 in, 2 out]
        n390 = Preview Queue Element(queue=w1173, timeout in ms (-1)=0, error in (no error)=w1174) -> (queue out=w1172:refnum<queue>, element=w1177:T6, error out=w1171:errorcluster)  [unwired: 1 out]
        n391 = Not Equal?(x=T6 "Busy" ("Cmd"), y=w1177) -> (x != y?=w1170:bool)
        n392 = case shown="True" w1170 {
          tunnel: [w1182 w1196] -> w1179
          tunnel: [w1181 w1195] -> w1178
          tunnel: w1172 -> [w1182 w1193]
          tunnel: w1171 -> [w1181 w1192]
          tunnel: [TRUE FALSE] -> w1169
          frame False {
          }
          frame True {
            n393 = local write "ACK 1"(FALSE ("ACK 1")) -> ()
            n394 = local write "ACK 5"(FALSE ("ACK 8")) -> ()
            n395 = local write "ACK 2"(FALSE ("ACK 6")) -> ()
            n396 = local write "ACK 6"(FALSE ("ACK 6")) -> ()
            n397 = local write "ACK 3"(FALSE ("ACK 8")) -> ()
            n398 = local write "ACK 7"(FALSE ("ACK 6")) -> ()
            n399 = Enqueue Element(queue=w1193, element=T6 "Exit" ("Cmd"), error in (no error)=w1192) -> (queue out=w1196:refnum<queue>, error out=w1195:errorcluster)  [unwired: 1 in, 1 out]
            n400 = local write "ACK 4"(FALSE ("Done")) -> ()
            n401 = local write "ACK 8"(FALSE ("Done")) -> ()
          }
        }
      }
      event "Reset": Value Change {
        # "only queue msg if not busy"
        n402 = event-data() -> ()  [unwired: 1 in, 2 out]
        n403 = Preview Queue Element(queue=w1201, timeout in ms (-1)=0, error in (no error)=w1200) -> (queue out=w1204:refnum<queue>, element=w1207:T6, error out=w1203:errorcluster)  [unwired: 1 out]
        n404 = Not Equal?(x=T6 "Busy" ("Cmd"), y=w1207) -> (x != y?=w1205:bool)
        n405 = case shown="True" w1205 {
          tunnel: w1204 -> [w1209 w1247]
          tunnel: w1203 -> [w1208 w1246]
          tunnel: [w1209 w1217] -> w1198
          tunnel: [w1208 w1218] -> w1199
          frame False {
          }
          frame True {
            n406 = Enqueue Element(queue=w1247, element=T6 "R" ("Cmd"), error in (no error)=w1246) -> (queue out=w1235:refnum<queue>, error out=w1234:errorcluster)  [unwired: 1 in, 1 out]
            n407 = local write "ACK 1"(FALSE ("ACK 1")) -> ()
            n408 = local write "ACK 5"(FALSE ("ACK 8")) -> ()
            n409 = Enqueue Element(queue=w1235, element=T6 "F" ("Cmd"), error in (no error)=w1234) -> (queue out=w1243:refnum<queue>, error out=w1233:errorcluster)  [unwired: 1 in, 1 out]
            n410 = local write "ACK 2"(FALSE ("ACK 6")) -> ()
            n411 = local write "ACK 6"(FALSE ("ACK 6")) -> ()
            n412 = Enqueue Element(queue=w1243, element=T6 "A" ("Cmd"), error in (no error)=w1233) -> (queue out=w1225:refnum<queue>, error out=w1224:errorcluster)  [unwired: 1 in, 1 out]
            n413 = Enqueue Element(queue=w1225, element=T6 "T" ("Cmd"), error in (no error)=w1224) -> (queue out=w1227:refnum<queue>, error out=w1226:errorcluster)  [unwired: 1 in, 1 out]
            n414 = local write "ACK 3"(FALSE ("ACK 8")) -> ()
            n415 = local write "ACK 7"(FALSE ("ACK 6")) -> ()
            n416 = Enqueue Element(queue=w1227, element=T6 "t" ("Cmd"), error in (no error)=w1226) -> (queue out=w1223:refnum<queue>, error out=w1222:errorcluster)  [unwired: 1 in, 1 out]
            n417 = local write "ACK 4"(FALSE ("Done")) -> ()
            n418 = Enqueue Element(queue=w1223, element=T6 "M" ("Cmd"), error in (no error)=w1222) -> (queue out=w1239:refnum<queue>, error out=w1232:errorcluster)  [unwired: 1 in, 1 out]
            n419 = Enqueue Element(queue=w1239, element=T6 "G" ("Cmd"), error in (no error)=w1232) -> (queue out=w1240:refnum<queue>, error out=w1231:errorcluster)  [unwired: 1 in, 1 out]
            n420 = Enqueue Element(queue=w1240, element=T6 "g" ("Cmd"), error in (no error)=w1231) -> (queue out=w1236:refnum<queue>, error out=w1230:errorcluster)  [unwired: 1 in, 1 out]
            n421 = Enqueue Element(queue=w1236, element=T6 "EEPROM_Pconsts" ("Cmd"), error in (no error)=w1230) -> (queue out=w1220:refnum<queue>, error out=w1219:errorcluster)  [unwired: 1 in, 1 out]
            n422 = Enqueue Element(queue=w1220, element=T6 "C" ("Cmd"), error in (no error)=w1219) -> (queue out=w1217:refnum<queue>, error out=w1218:errorcluster)  [unwired: 1 in, 1 out]
          }
        }
      }
      event "Start streaming": Value Change {
        # "only queue msg if not busy AND main power is on"
        n423 = event-data() -> ()  [unwired: 1 in, 2 out]
        n424 = local read "System status"() -> (w1250:T4)
        n425 = Unbundle By Name(w1250) -> ("Main power"=w1249:bool)
        n426 = Preview Queue Element(queue=w1256, timeout in ms (-1)=0, error in (no error)=w1253) -> (queue out=w1259:refnum<queue>, element=w1262:T6, error out=w1258:errorcluster)  [unwired: 1 out]
        n427 = Not Equal?(x=T6 "Busy" ("Cmd"), y=w1262) -> (x != y?=w1260:bool)
        n428 = And(x=w1249, y=w1260) -> (x .and. y?=w1251:bool)
        n429 = case shown="True" w1251 {
          tunnel: w1259 -> [w1264 w1268]
          tunnel: w1258 -> [w1263 w1267]
          tunnel: [w1264 w1265] -> w1255
          tunnel: [w1263 w1266] -> w1254
          frame False {
          }
          frame True {
            n430 = Enqueue Element(queue=w1268, element=T6 "S" ("Cmd"), error in (no error)=w1267) -> (queue out=w1265:refnum<queue>, error out=w1266:errorcluster)  [unwired: 1 in, 1 out]
          }
        }
      }
      event "Apply settings 1": Value Change {
        # "only queue msg if not busy"
        n431 = event-data() -> ()  [unwired: 1 in, 2 out]
        n432 = Preview Queue Element(queue=w1274, timeout in ms (-1)=0, error in (no error)=w1273) -> (queue out=w1277:refnum<queue>, element=w1280:T6, error out=w1276:errorcluster)  [unwired: 1 out]
        n433 = Not Equal?(x=T6 "Busy" ("Cmd"), y=w1280) -> (x != y?=w1278:bool)
        n434 = case shown="True" w1278 {
          tunnel: w1277 -> [w1282 w1296]
          tunnel: w1276 -> [w1281 w1295]
          tunnel: [w1282 w1285] -> w1270
          tunnel: [w1281 w1284] -> w1271
          frame False {
          }
          frame True {
            n435 = local write "ACK 2"(FALSE ("ACK 1")) -> ()
            n436 = Enqueue Element(queue=w1296, element=T6 "T" ("Cmd"), error in (no error)=w1295) -> (queue out=w1293:refnum<queue>, error out=w1292:errorcluster)  [unwired: 1 in, 1 out]
            n437 = Enqueue Element(queue=w1293, element=T6 "t" ("Cmd"), error in (no error)=w1292) -> (queue out=w1290:refnum<queue>, error out=w1291:errorcluster)  [unwired: 1 in, 1 out]
            n438 = Enqueue Element(queue=w1290, element=T6 "M" ("Cmd"), error in (no error)=w1291) -> (queue out=w1287:refnum<queue>, error out=w1286:errorcluster)  [unwired: 1 in, 1 out]
            n439 = Enqueue Element(queue=w1287, element=T6 "g" ("Cmd"), error in (no error)=w1286) -> (queue out=w1285:refnum<queue>, error out=w1284:errorcluster)  [unwired: 1 in, 1 out]
          }
        }
      }
      event "Apply settings 2": Value Change {
        # "only queue msg if not busy"
        n440 = event-data() -> ()  [unwired: 1 in, 2 out]
        n441 = Preview Queue Element(queue=w1302, timeout in ms (-1)=0, error in (no error)=w1301) -> (queue out=w1305:refnum<queue>, element=w1308:T6, error out=w1304:errorcluster)  [unwired: 1 out]
        n442 = Not Equal?(x=T6 "Busy" ("Cmd"), y=w1308) -> (x != y?=w1306:bool)
        n443 = case shown="True" w1306 {
          tunnel: w1305 -> [w1310 w1330]
          tunnel: w1304 -> [w1309 w1329]
          tunnel: [w1310 w1311] -> w1299
          tunnel: [w1309 w1312] -> w1300
          frame False {
          }
          frame True {
            n444 = local write "ACK 3"(FALSE ("ACK 1")) -> ()
            n445 = Enqueue Element(queue=w1330, element=T6 "O" ("Cmd"), error in (no error)=w1329) -> (queue out=w1326:refnum<queue>, error out=w1325:errorcluster)  [unwired: 1 in, 1 out]
            n446 = Enqueue Element(queue=w1326, element=T6 "G" ("Cmd"), error in (no error)=w1325) -> (queue out=w1314:refnum<queue>, error out=w1313:errorcluster)  [unwired: 1 in, 1 out]
            n447 = Enqueue Element(queue=w1314, element=T6 "F" ("Cmd"), error in (no error)=w1313) -> (queue out=w1318:refnum<queue>, error out=w1319:errorcluster)  [unwired: 1 in, 1 out]
            n448 = Enqueue Element(queue=w1318, element=T6 "A" ("Cmd"), error in (no error)=w1319) -> (queue out=w1316:refnum<queue>, error out=w1315:errorcluster)  [unwired: 1 in, 1 out]
            n449 = Enqueue Element(queue=w1316, element=T6 "M" ("Cmd"), error in (no error)=w1315) -> (queue out=w1323:refnum<queue>, error out=w1324:errorcluster)  [unwired: 1 in, 1 out]
            n450 = Enqueue Element(queue=w1323, element=T6 "EEPROM_Pconsts" ("Cmd"), error in (no error)=w1324) -> (queue out=w1311:refnum<queue>, error out=w1312:errorcluster)  [unwired: 1 in, 1 out]
          }
        }
      }
      event "Refresh sys. status": Value Change {
        # "only queue msg if not busy"
        n451 = event-data() -> ()  [unwired: 1 in, 2 out]
        n452 = Preview Queue Element(queue=w1336, timeout in ms (-1)=0, error in (no error)=w1335) -> (queue out=w1339:refnum<queue>, element=w1342:T6, error out=w1338:errorcluster)  [unwired: 1 out]
        n453 = Not Equal?(x=T6 "Busy" ("Cmd"), y=w1342) -> (x != y?=w1340:bool)
        n454 = case shown="True" w1340 {
          tunnel: w1339 -> [w1344 w1352]
          tunnel: w1338 -> [w1343 w1351]
          tunnel: [w1344 w1349] -> w1334
          tunnel: [w1343 w1348] -> w1333
          frame False {
          }
          frame True {
            n455 = local write "ACK 5"(FALSE ("ACK 1")) -> ()
            n456 = Enqueue Element(queue=w1352, element=T6 "G" ("Cmd"), error in (no error)=w1351) -> (queue out=w1350:refnum<queue>, error out=w1347:errorcluster)  [unwired: 1 in, 1 out]
            n457 = Enqueue Element(queue=w1350, element=T6 "g" ("Cmd"), error in (no error)=w1347) -> (queue out=w1349:refnum<queue>, error out=w1348:errorcluster)  [unwired: 1 in, 1 out]
          }
        }
      }
      event "Apply settings 3": Value Change {
        # "only queue msg if not busy"
        n458 = event-data() -> ()  [unwired: 1 in, 2 out]
        n459 = Preview Queue Element(queue=w1358, timeout in ms (-1)=0, error in (no error)=w1357) -> (queue out=w1361:refnum<queue>, element=w1364:T6, error out=w1360:errorcluster)  [unwired: 1 out]
        n460 = Not Equal?(x=T6 "Busy" ("Cmd"), y=w1364) -> (x != y?=w1362:bool)
        n461 = case shown="True" w1362 {
          tunnel: w1361 -> [w1366 w1371]
          tunnel: w1360 -> [w1365 w1370]
          tunnel: [w1366 w1368] -> w1355
          tunnel: [w1365 w1369] -> w1356
          frame False {
          }
          frame True {
            n462 = local write "ACK 4"(FALSE ("ACK 1")) -> ()
            n463 = Enqueue Element(queue=w1371, element=T6 "C" ("Cmd"), error in (no error)=w1370) -> (queue out=w1368:refnum<queue>, error out=w1369:errorcluster)  [unwired: 1 in, 1 out]
          }
        }
      }
      event "Write ASCII datalog": Value Change {
        # "only queue msg if not busy"
        n464 = event-data() -> ()  [unwired: 1 in, 2 out]
        n465 = Preview Queue Element(queue=w1377, timeout in ms (-1)=0, error in (no error)=w1376) -> (queue out=w1380:refnum<queue>, element=w1383:T6, error out=w1379:errorcluster)  [unwired: 1 out]
        n466 = Not Equal?(x=T6 "Busy" ("Cmd"), y=w1383) -> (x != y?=w1381:bool)
        n467 = case shown="True" w1381 {
          tunnel: w1380 -> [w1385 w1389]
          tunnel: w1379 -> [w1384 w1388]
          tunnel: [w1385 w1386] -> w1375
          tunnel: [w1384 w1387] -> w1374
          frame False {
          }
          frame True {
            n468 = local write "ASCII done"(FALSE ("ACK 1")) -> ()
            n469 = Enqueue Element(queue=w1389, element=T6 "convert_datalogs" ("Cmd"), error in (no error)=w1388) -> (queue out=w1386:refnum<queue>, error out=w1387:errorcluster)  [unwired: 1 in, 1 out]
          }
        }
      }
    }
  }
  n470 = Merge Errors(w32, w30) -> (w33:errorcluster)
  n471 = Release Queue(queue=w31, error in (no error)=w33) -> (error out=w17:errorcluster)  [unwired: 1 in, 2 out]
  n472 = Merge Errors(w17, w18) -> (w19:errorcluster)
  n473 = local write "Error"(w19) -> ()
